vi "Two Parameter Marco Reparam.vi"() -> ()   [LabVIEW 2015]
uses:
  <vilib>/Platform/TimedLoop/XDataNode/timing_clust.ctl
  <vilib>/Platform/TimedLoop/XDataNode/nitl_modes.ctl
  <vilib>/Platform/TimedLoop/XDataNode/wakeup.ctl
  <vilib>/DAQmx/read.llb/DAQmx Read (Analog DBL 1Chan 1Samp).vi
  <vilib>/DAQmx/read.llb/DAQmx Read (Analog 1D DBL NChan 1Samp).vi
  <vilib>/DAQmx/create/channels.llb/DAQmx Create Channel (AI-Voltage-Basic).vi
  <vilib>/Enthought/Python Integration Toolkit/api/Unpack Double.vi
  <vilib>/DAQmx/miscellaneous.llb/DAQmx Fill In Error Info.vi
  <vilib>/Platform/TimedLoop/XDataNode/XDataNode.xnode
  Program Files/neMESYS_SDK/neMESYS LabVIEW Kit/neMESYS LabVIEW Integration Kit.lvlib
  <vilib>/Platform/TimedLoop/XDataNode/XDNodeRunTimeDep.lvlib
  Conor/Temp CN7500/Omega CN7500/Omega CN7500.lvlib
  <vilib>/Enthought/Python Integration Toolkit/Python Integration Toolkit.lvlib
panel:
  in  "LogFileName must end with .txt":string
  out "Param 1 8":dbl
  out "T value 1 8":dbl
  out "Param 2 8":dbl
  out "T value 2 8":dbl
  out "T Ref 8":dbl
  out "Correlation 8":dbl
  out "X2 8":dbl
  out "X2 ref 8":dbl
  out "Temp 9":dbl
  out "Flow 9":dbl
  out "Conc 9":dbl
  out "C BAcid 8":dbl
  out "C EB 8":dbl
  out "Exp 9":bool
  out "Param 1 7":dbl
  out "T value 1 7":dbl
  out "Param 2 7":dbl
  out "T value 2 7":dbl
  out "T Ref 7":dbl
  out "Correlation 7":dbl
  out "X2 7":dbl
  out "X2 ref 7":dbl
  out "Temp 8":dbl
  out "Flow 8":dbl
  out "Conc 8":dbl
  out "C BAcid 7":dbl
  out "C EB 7":dbl
  out "Exp 8":bool
  out "Param 1 6":dbl
  out "T value 1 6":dbl
  out "Param 2 6":dbl
  out "T value 2 6":dbl
  out "T Ref 6":dbl
  out "Correlation 6":dbl
  out "X2 6":dbl
  out "X2 ref 6":dbl
  out "Temp 7":dbl
  out "Flow 7":dbl
  out "Conc 7":dbl
  out "C BAcid 6":dbl
  out "C EB 6":dbl
  out "Exp 7":bool
  out "Param 1 5":dbl
  out "T value 1 5":dbl
  out "Param 2 5":dbl
  out "T value 2 5":dbl
  out "T Ref 5":dbl
  out "Correlation 5":dbl
  out "X2 5":dbl
  out "X2 ref 5":dbl
  out "Temp 6":dbl
  out "Flow 6":dbl
  out "Conc 6":dbl
  out "C BAcid 5":dbl
  out "C EB 5":dbl
  out "Exp 6":bool
  out "Param 1 4":dbl
  out "T value 1 4":dbl
  out "Param 2 4":dbl
  out "T value 2 4":dbl
  out "T Ref 4":dbl
  out "Correlation 4":dbl
  out "X2 4":dbl
  out "X2 ref 4":dbl
  out "Temp 5":dbl
  out "Flow 5":dbl
  out "Conc 5":dbl
  out "C BAcid 4":dbl
  out "C EB 4":dbl
  out "Exp 5":bool
  out "Param 1 3":dbl
  out "T value 1 3":dbl
  out "Param 2 3":dbl
  out "T value 2 3":dbl
  out "T Ref 3":dbl
  out "Correlation 3":dbl
  out "X2 3":dbl
  out "X2 ref 3":dbl
  out "Temp 4":dbl
  out "Flow 4":dbl
  out "Conc 4":dbl
  out "C BAcid 3":dbl
  out "C EB 3":dbl
  out "Exp 4":bool
  out "Conc 3":dbl
  out "Flow 3":dbl
  out "Temp 3":dbl
  in  "Design Criteria A or D or E or SV":string
  in  "Reparameterise? ON or OFF":string
  out "Exp 2":bool
  out "C EB 1":dbl
  out "C BAcid 1":dbl
  out "X2 ref 2":dbl
  out "X2 2":dbl
  out "Exp 2":bool
  out "Liquid Inlet Pressure (bar g)":dbl
  in  "Liquid P sensor Terminal Configuration":i32(ring)=-1 items=["default"=-1, "RSE"=10083, "NRSE"=10078, "Differential"=10106, "Pseudodifferential"=12529]
  in  "Liquid P sensor Physical Channel":tag="Dev1/ai0"
  in  "Temp 2":dbl
  in  "Conc 2":dbl
  in  "Flow 2":dbl
  out "Correlation 2":dbl
  out "T Ref 2":dbl
  out "Exp 3":bool
  out "Exp 1":bool
  out "Exp 0":bool
  out "Conc 1":dbl
  out "Flow 1":dbl
  out "Temp 1":dbl
  out "Conc 2":dbl
  out "Flow 2":dbl
  out "Temp 2":dbl
  out "Param 1 2":dbl
  out "T value 1 2":dbl
  out "Param 2 2":dbl
  out "T value 2 2":dbl
  out "C BAcid 2":dbl
  out "C EB 2":dbl
  in  "Result file name must end with .xlsx":string
  in  "HPLC file Name, dont need extension":string
  out "Desired Conc Not Possible":bool
  in  "Safety or Emergency Syringe Control":bool
  out "Feed Concentration (M)":dbl
  out "Total Flowrate (uL/min)":dbl
  out "Gas Back Pressure (barg)":dbl
  in  "Shut down in empty?\nLeft off, right on":bool
  in  "Clear":bool
  out "Safety Shut Down Pressure (barg)":dbl
  out "Calculated Pressure":dbl[](graph)
  out "Safety Shut Down Temp":dbl
  out "Actual Temp (oC)":dbl
  out "Temperature":dynamicdata(graph)
  out "Temp Set Point (oC)":dbl
  in  "Temp 1":dbl
  in  "Temp 0":dbl
  in  "Update Temperature Set Point":bool
  in  "Automated Experiments or Direct Control":bool
  in  "Set Point (oC)":dbl
  out "loop ind":dbl
  in  "Stop everything":bool
  in  "Skip Exp":bool
  in  "Minutes between Exp":dbl min=0.0 step=0.05
  in  "Refill 4":bool
  in  "Refill 3":bool
  in  "Refill 2":bool
  in  "Refill 1":bool
  in  "Empty 4":bool
  in  "Empty 3":bool
  in  "Empty 2":bool
  in  "Empty 1":bool
  in  "Calibrate 4":bool
  in  "Calibrate 3":bool
  in  "Calibrate 2":bool
  in  "Calibrate 1":bool
  in  "Stop Dose 4":bool
  in  "Stop Dose 3":bool
  in  "Stop Dose 2":bool
  in  "Stop Dose 1":bool
  in  "Flow 1":dbl
  in  "Conc 1":dbl
  in  "Flow 0":dbl
  in  "Conc 0":dbl
  in  "Generate Flow":bool
  in  "Set Flowrate 1":dbl
  in  "Set Flowrate 2":dbl
  in  "Set Flowrate 3":dbl
  in  "Set Flowrate 4":dbl
  in  "High Conc":dbl min=0.0 max=2.0
  in  "Low Conc":dbl min=0.0 max=2.0
  out "Volumetric Fraction Acid":dbl min=0.0 max=1.0
  out "Syringe Level 4":dbl(slide) scale=0.0..5500.0
  out "Syringe Level 3":dbl(slide) scale=0.0..5500.0
  out "Syringe Level 2":dbl(slide) scale=0.0..5500.0
  out "Syringe Level 1":dbl(slide) scale=0.0..5500.0
  out "Flowrate 4 Ethanol":dbl
  out "Flowrate 3 Acid":dbl
  out "Flowrate 2 High":dbl
  out "Flowrate 1 Low":dbl
  # "Pre Planned Experiments"
  # "Conducted Experiments Set Points"
  # "Safety (start and end)"
  # "Current Conditions"
  # "(uL/min)"
  # "Coerced to nearest possible"
  # "Experimental Info"
  # "Acid must be between 0 and 1, normally 0.1 for 10%"
  # "Direct Control"
  # "Unit of Gas Flow NmL/min"
  # "I swapped syringe 1 and 2, so now 2 is high and 1 is low"
  # "Emergency Syringe Control Below"
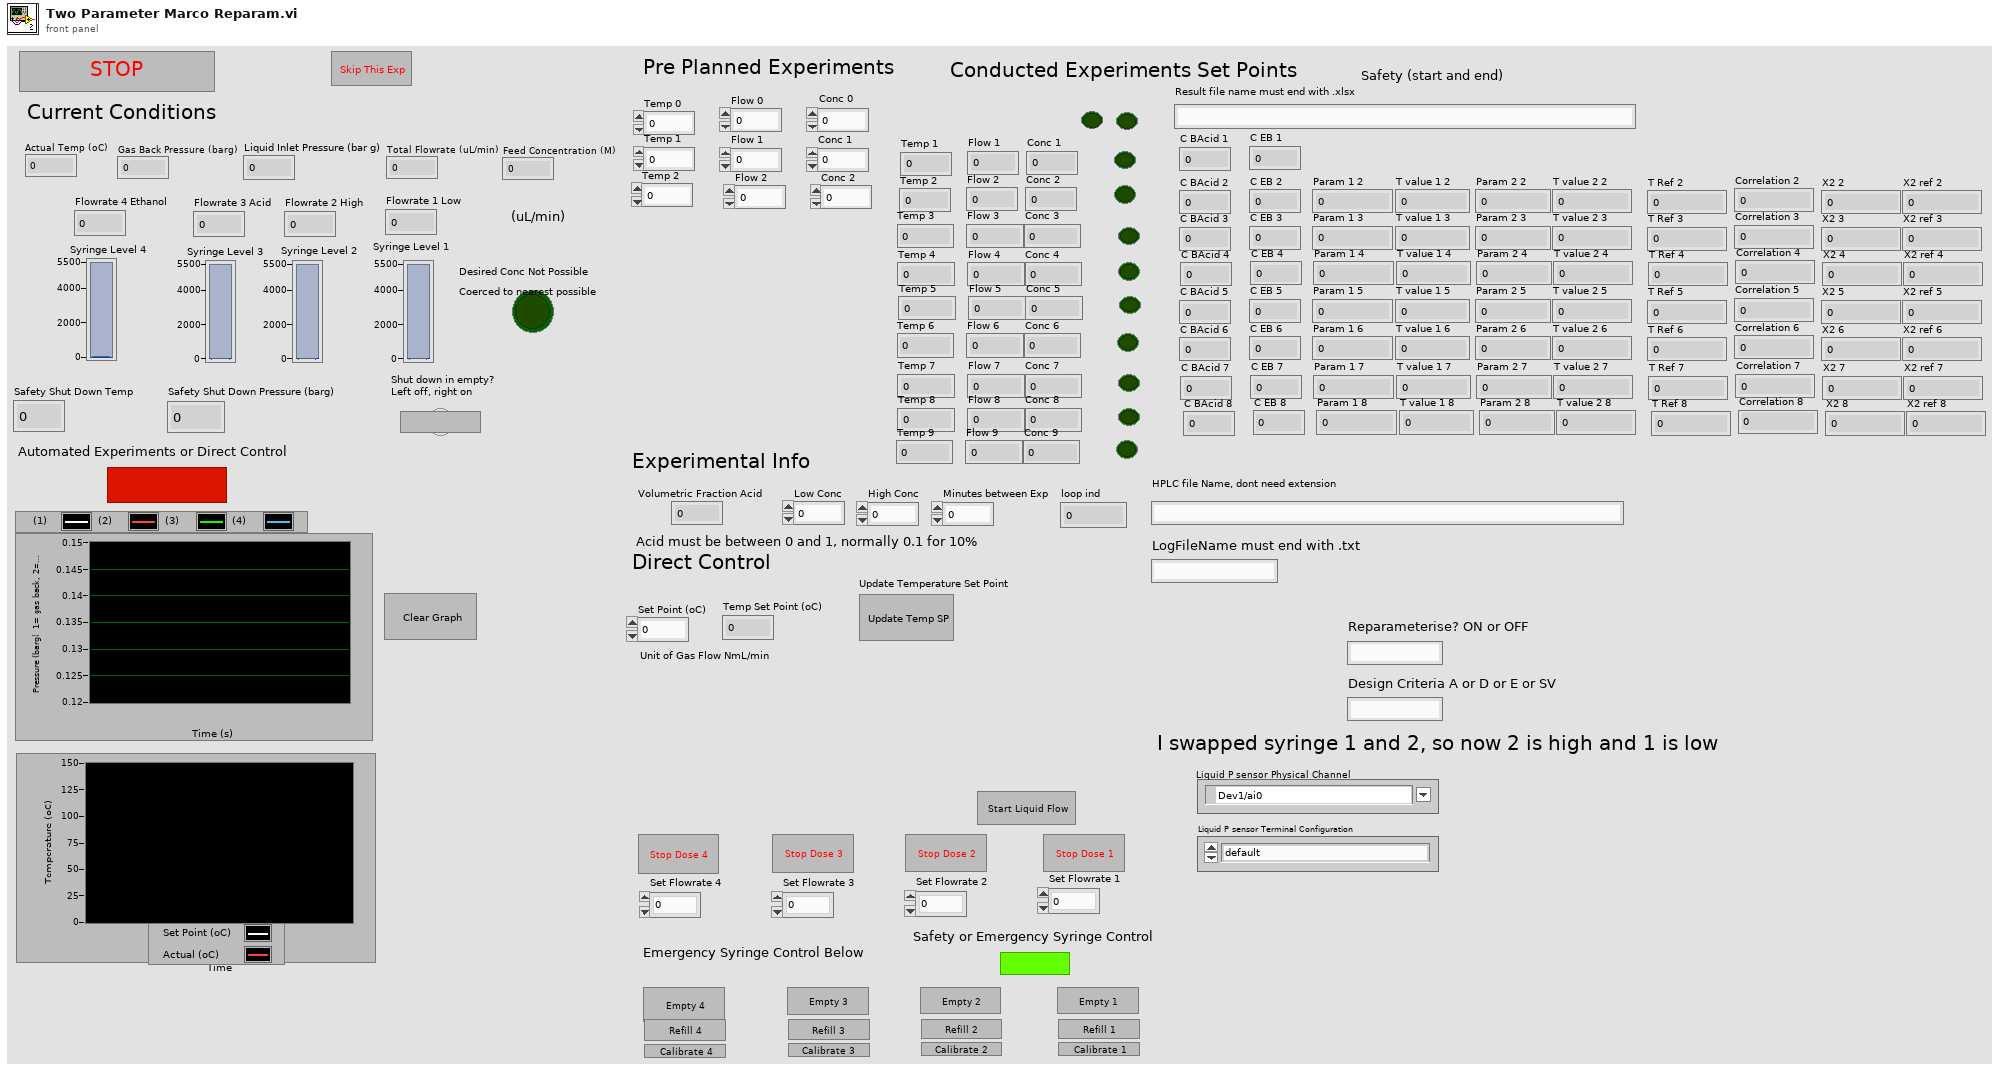
[diagram p1: front panel]
types:
  T1 = typedef "XDNodeRunTimeDep.lvlib/timing_clust.ctl" = cluster{"Expected End [f-1]":u64, "Actual End [f-1]":u64, "Finished Late? [f-1]":bool, "Expected End [i-1]":u64, "Actual End [i-1]":u64, "Finished Late? [i-1]":bool, "Expected Start [i]":u64, "Actual Start [i]":u64, "Expected Start [f]":u64, "Actual Start [f]":u64, "Source Name":string, "Structure Name":string, "Period":i64, "Deadline":i64, "Offset":i64, "Start":i64, "Priority":i32, "Timeout":i32, "Mode":T2, "Wakeup Reason":T3, "Error":errorcluster, "Source Type":string, "Secondary Source Type":string, "Global End Time":u64, "Global Start Time":u64, "Frame Duration":u64, "Iteration Duration":u64, "Assigned CPU":i32, "I/O Scan Engine Mode":u32}
  T2 = typedef "XDNodeRunTimeDep.lvlib/nitl_modes.ctl" = enum32{"No Change", "Process missed periods, maintain original phase", "Discard missed periods, maintain original phase", "Process missed periods, ignore original phase", "Discard missed periods, ignore original phase"}
  T3 = typedef "XDNodeRunTimeDep.lvlib/wakeup.ctl" = enum32{"Normal", "Aborted", "Asynchronous wakeup", "Timing source error", "Timed loop error", "Timeout"}
  T4 = typedef "Python Integration Toolkit.lvlib/Session ID.ctl" = u64
  T5 = typedef "Python Integration Toolkit.lvlib/Python Objects.ctl" = variant
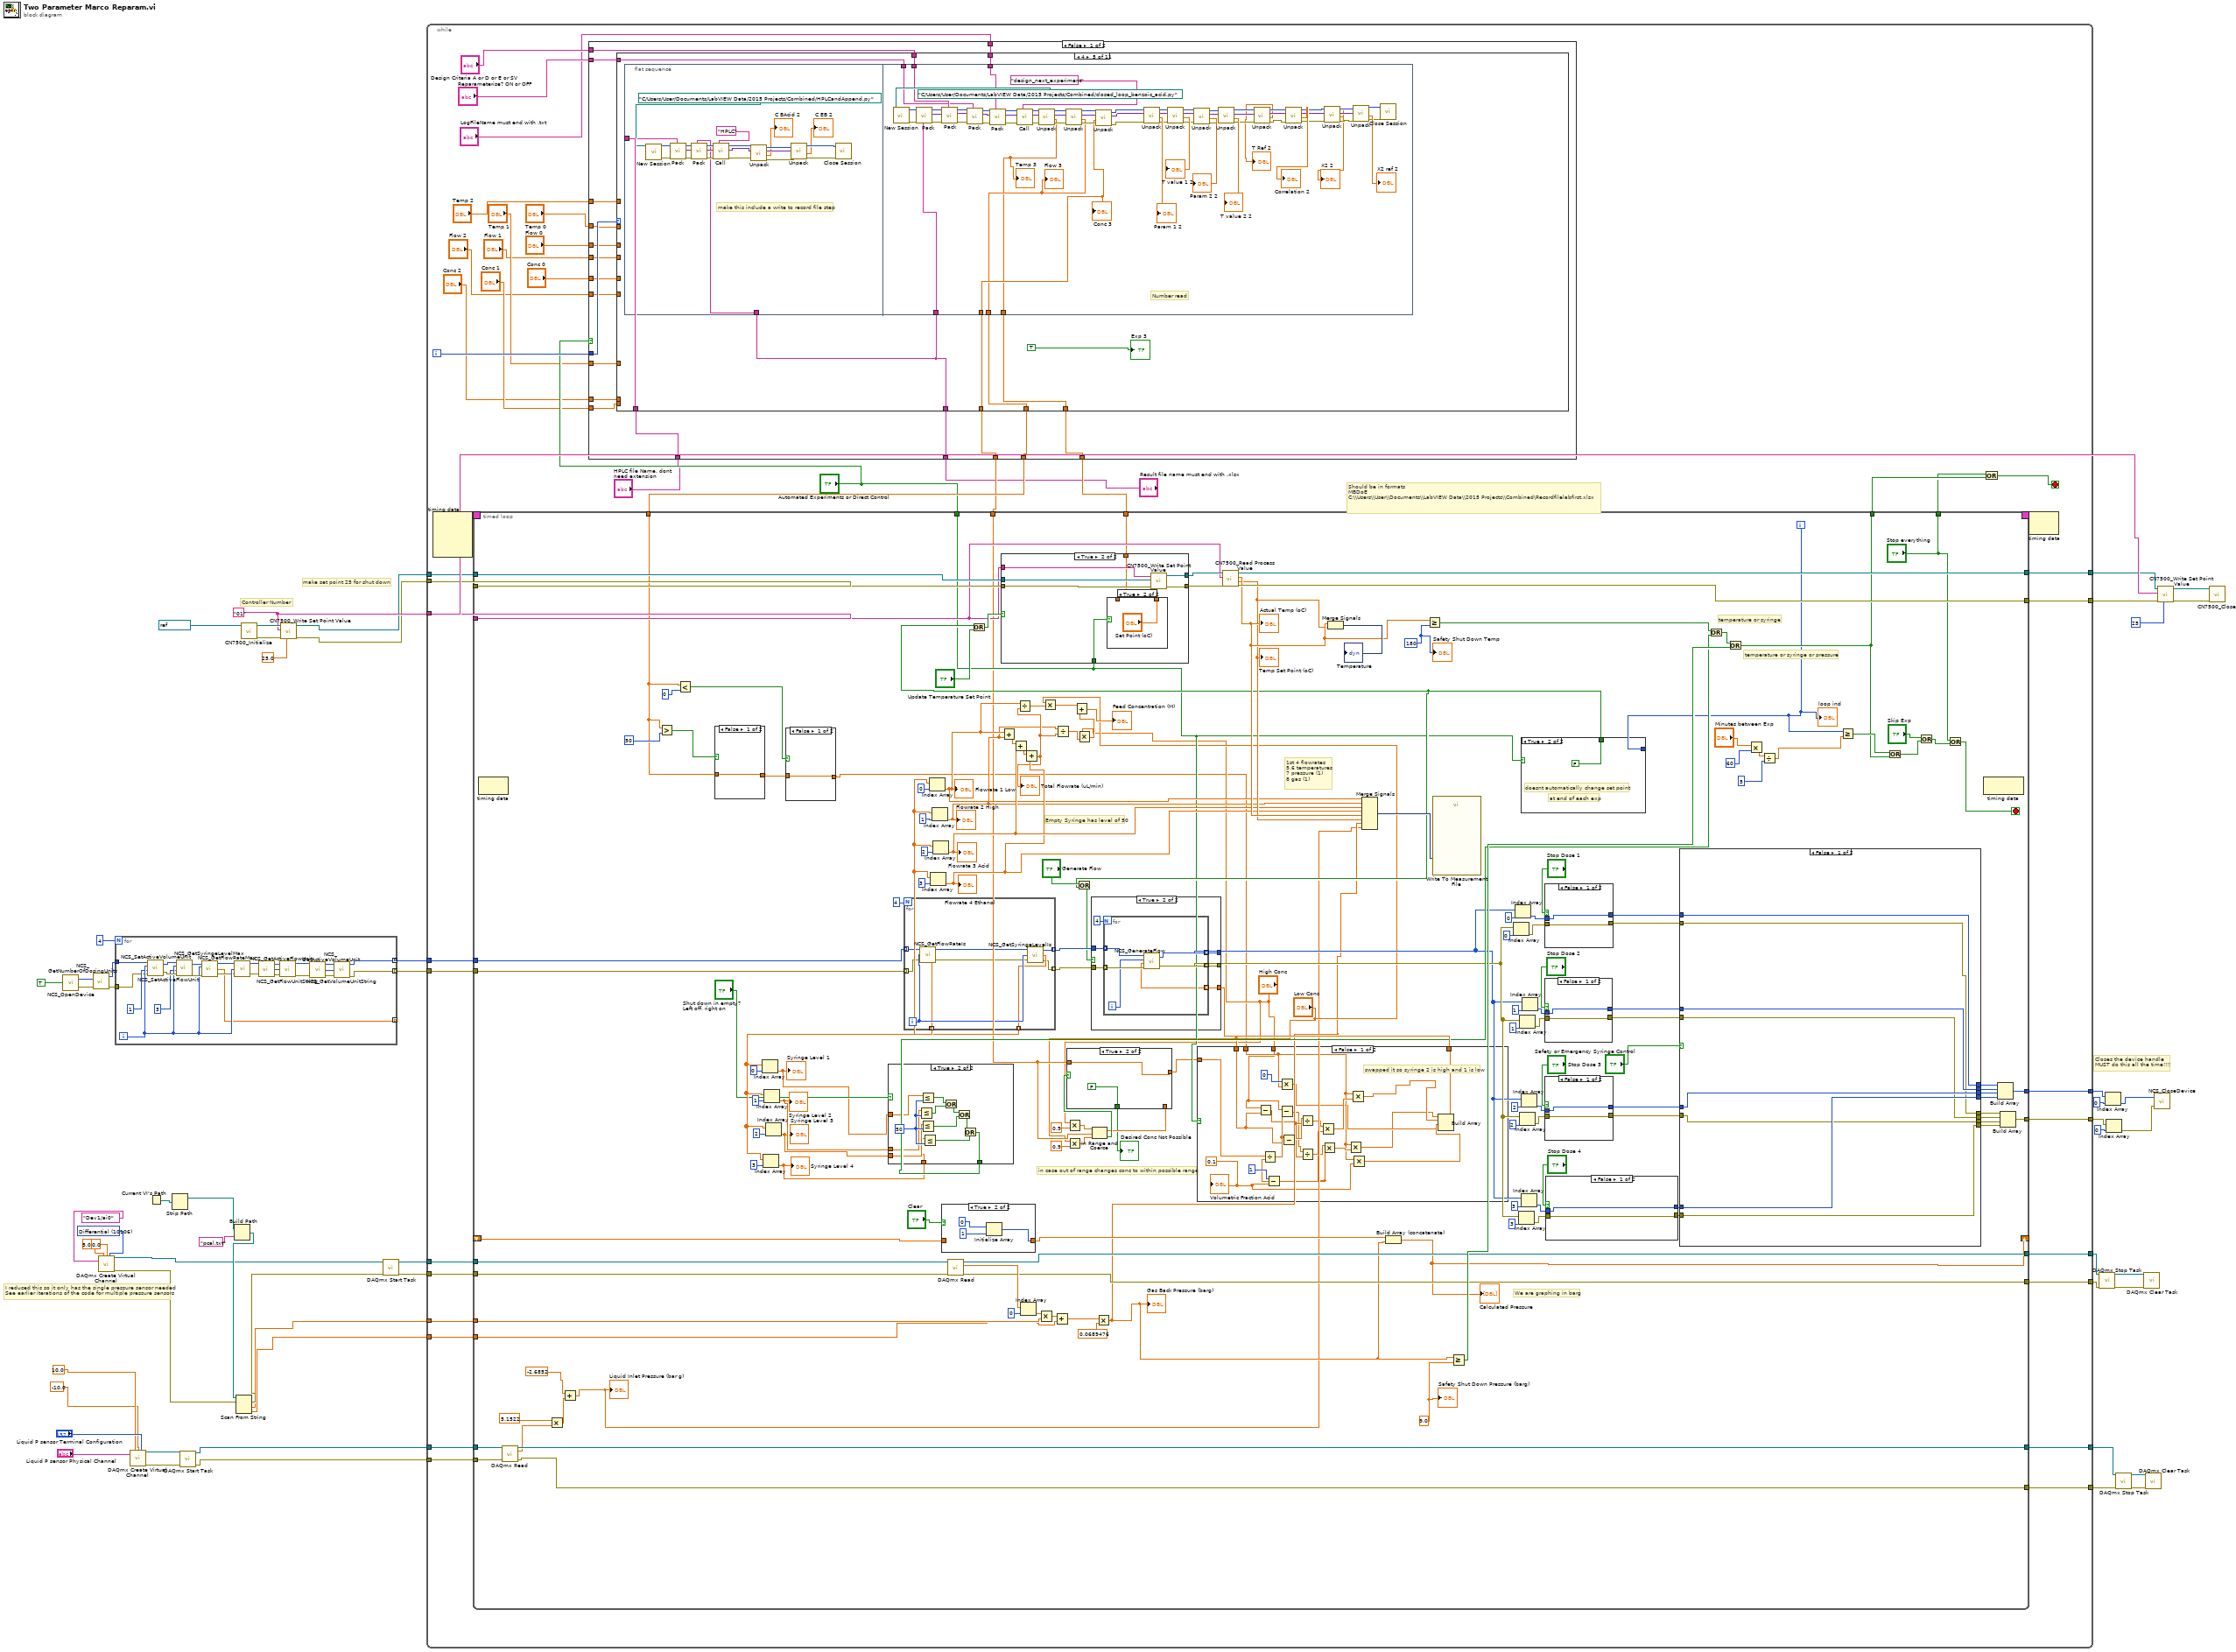
[diagram p0: block diagram]
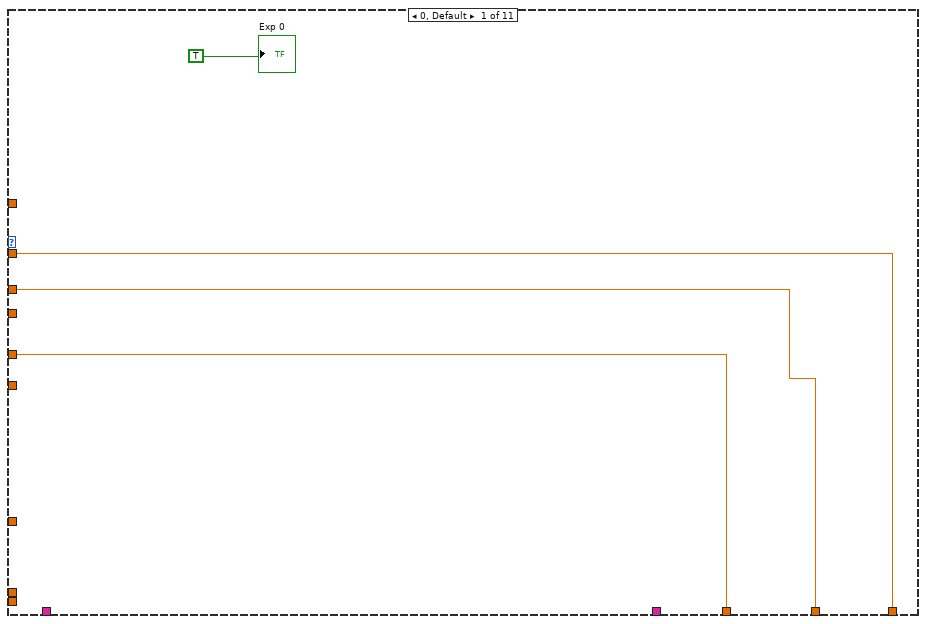
[diagram p2: hidden frame]
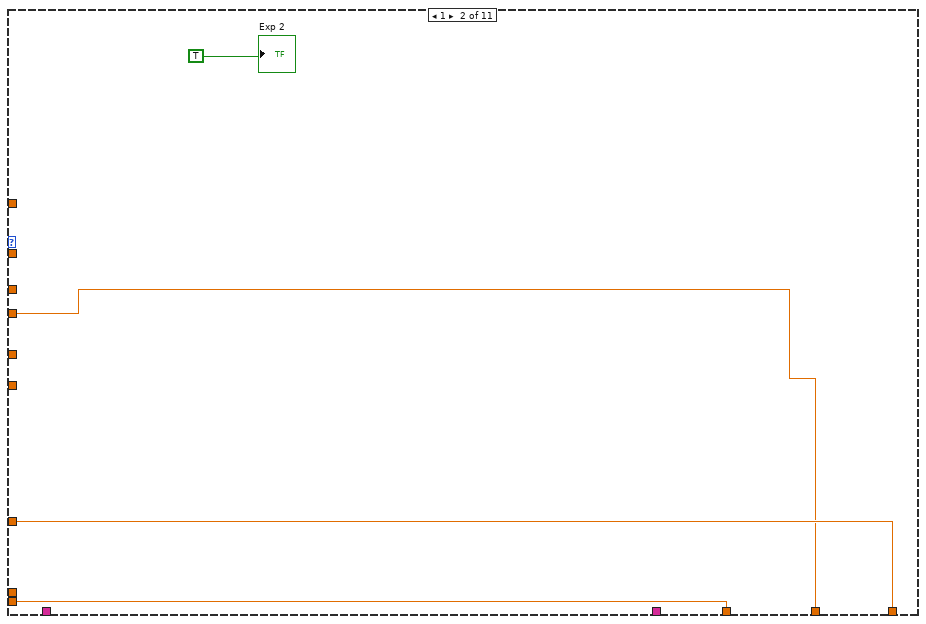
[diagram p3: hidden frame]
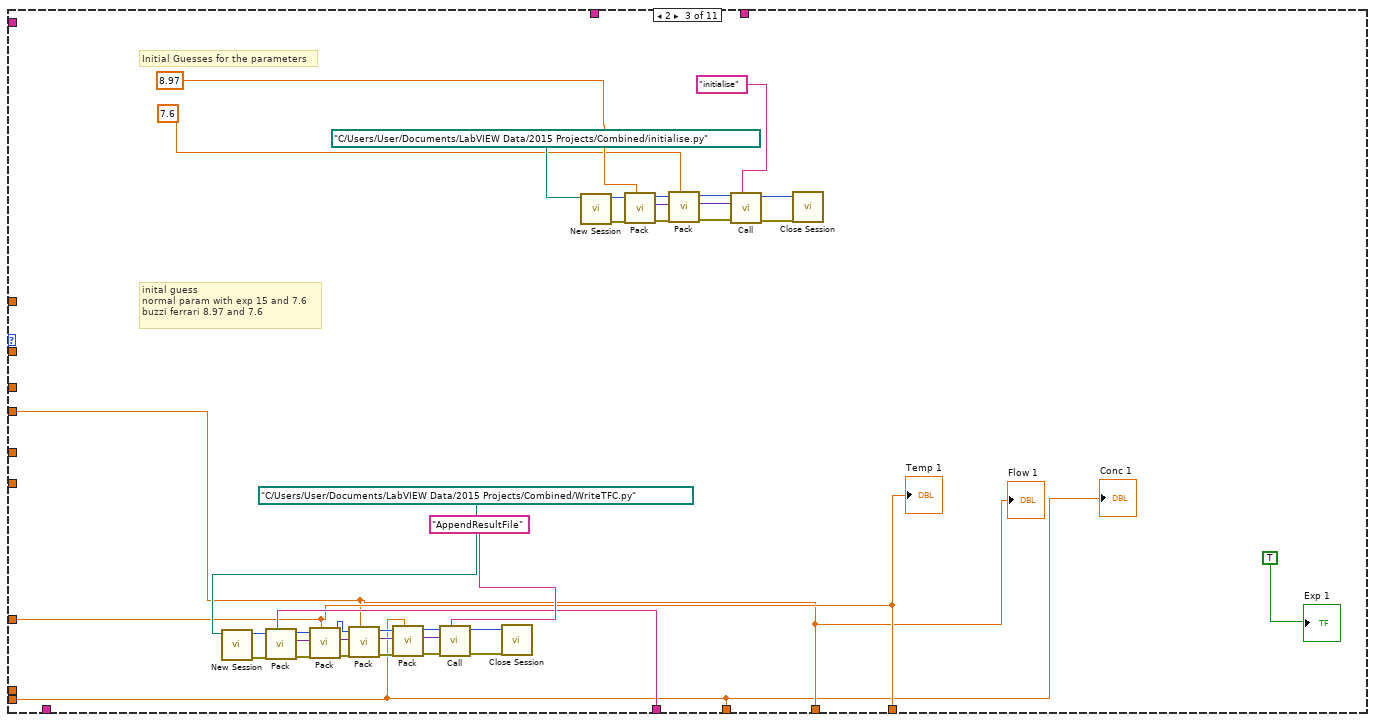
[diagram p4: hidden frame]
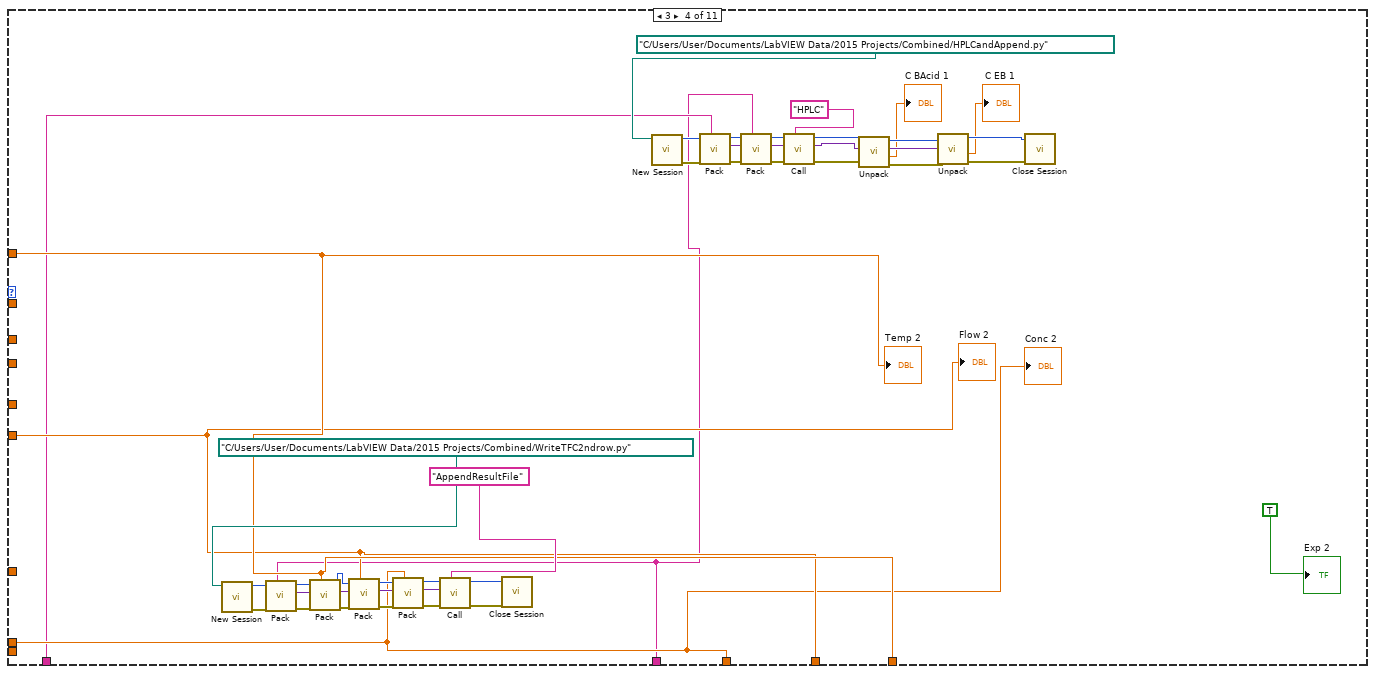
[diagram p5: hidden frame]
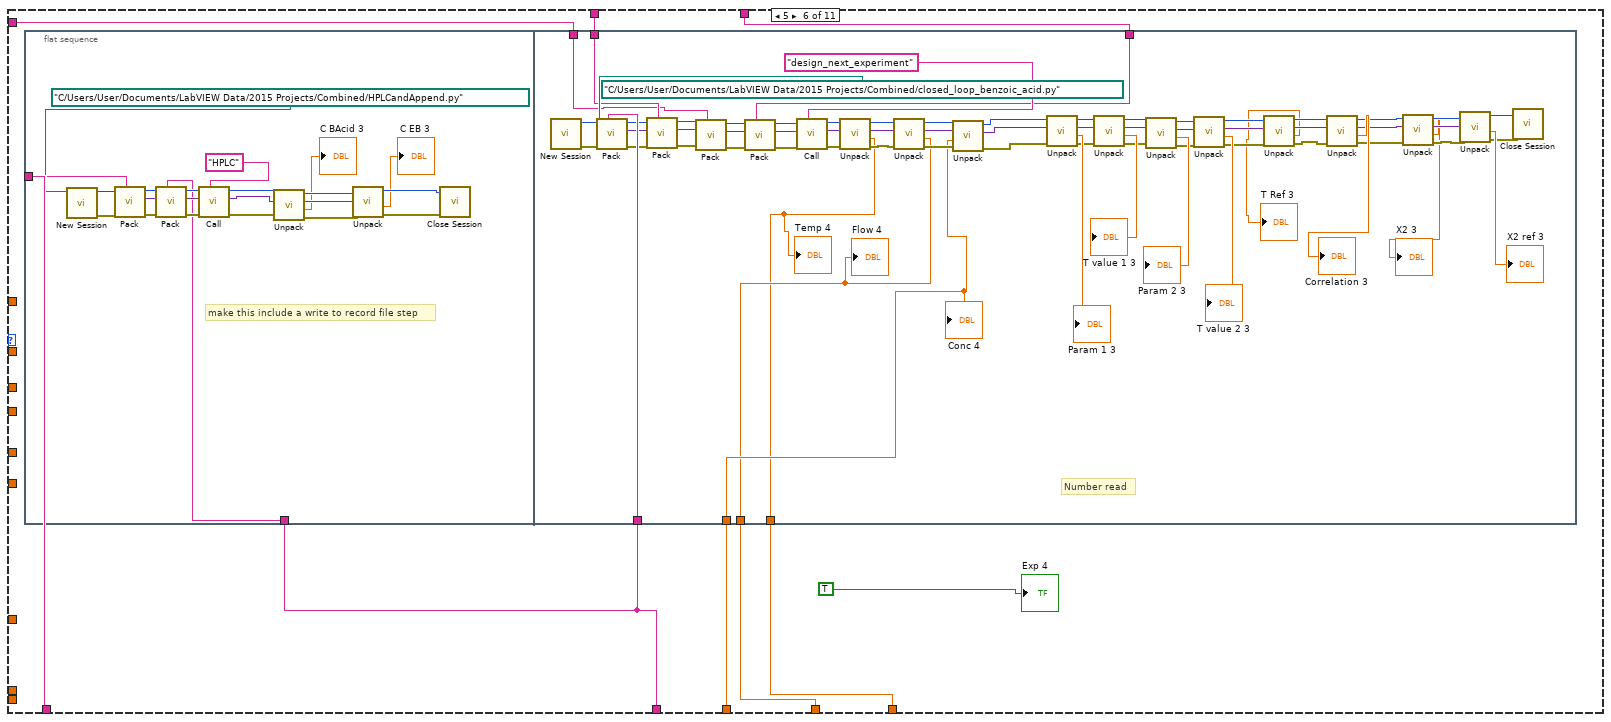
[diagram p6: hidden frame]
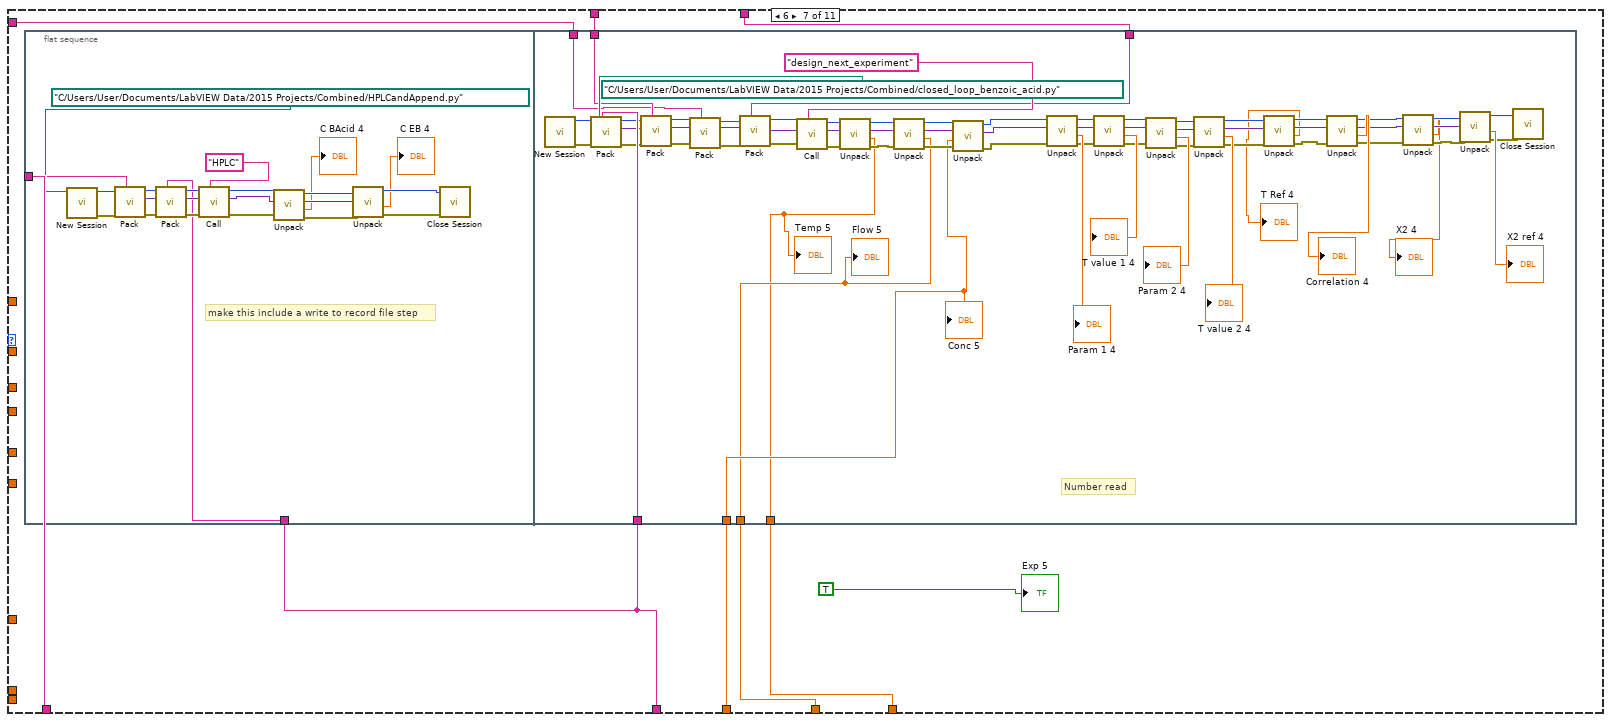
[diagram p7: hidden frame]
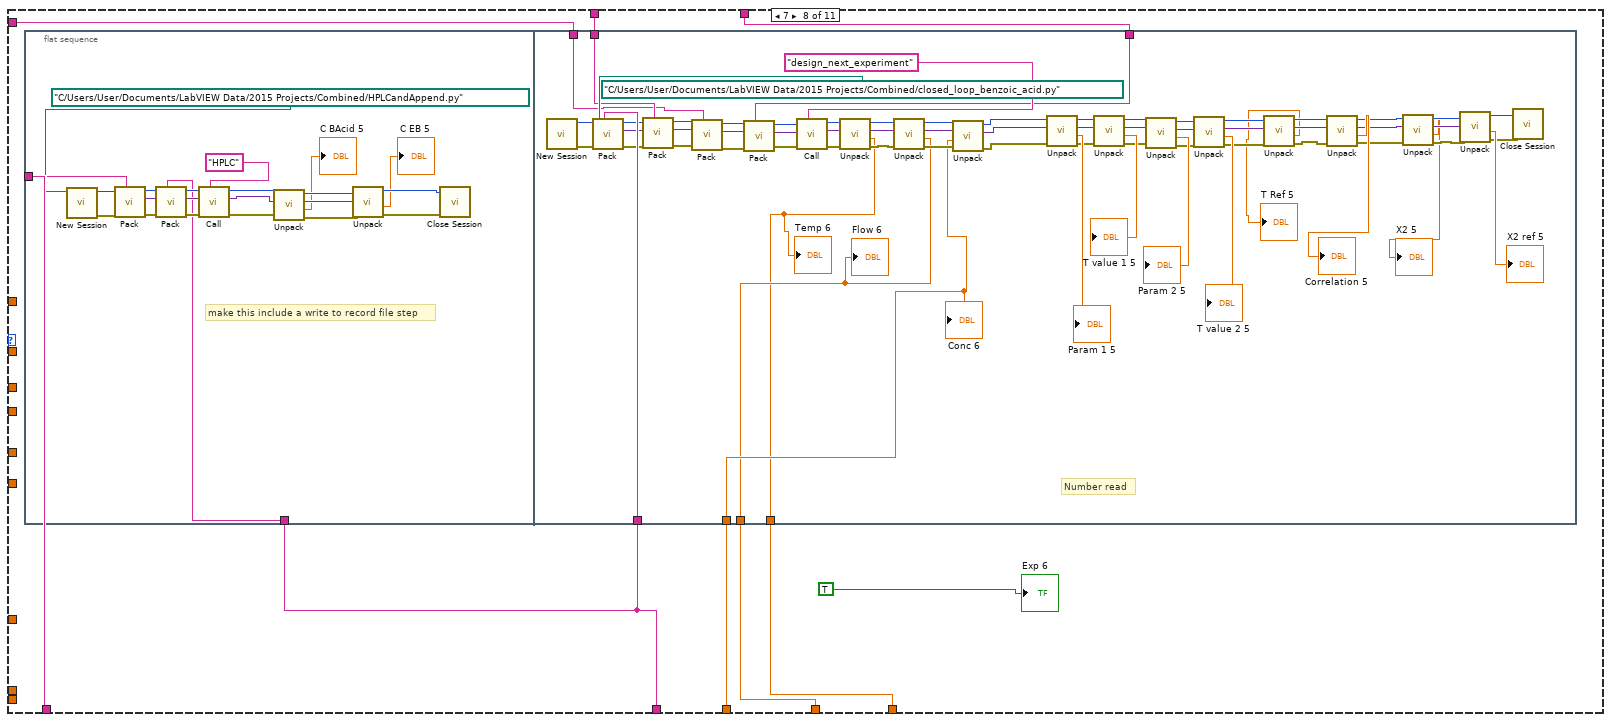
[diagram p8: hidden frame]
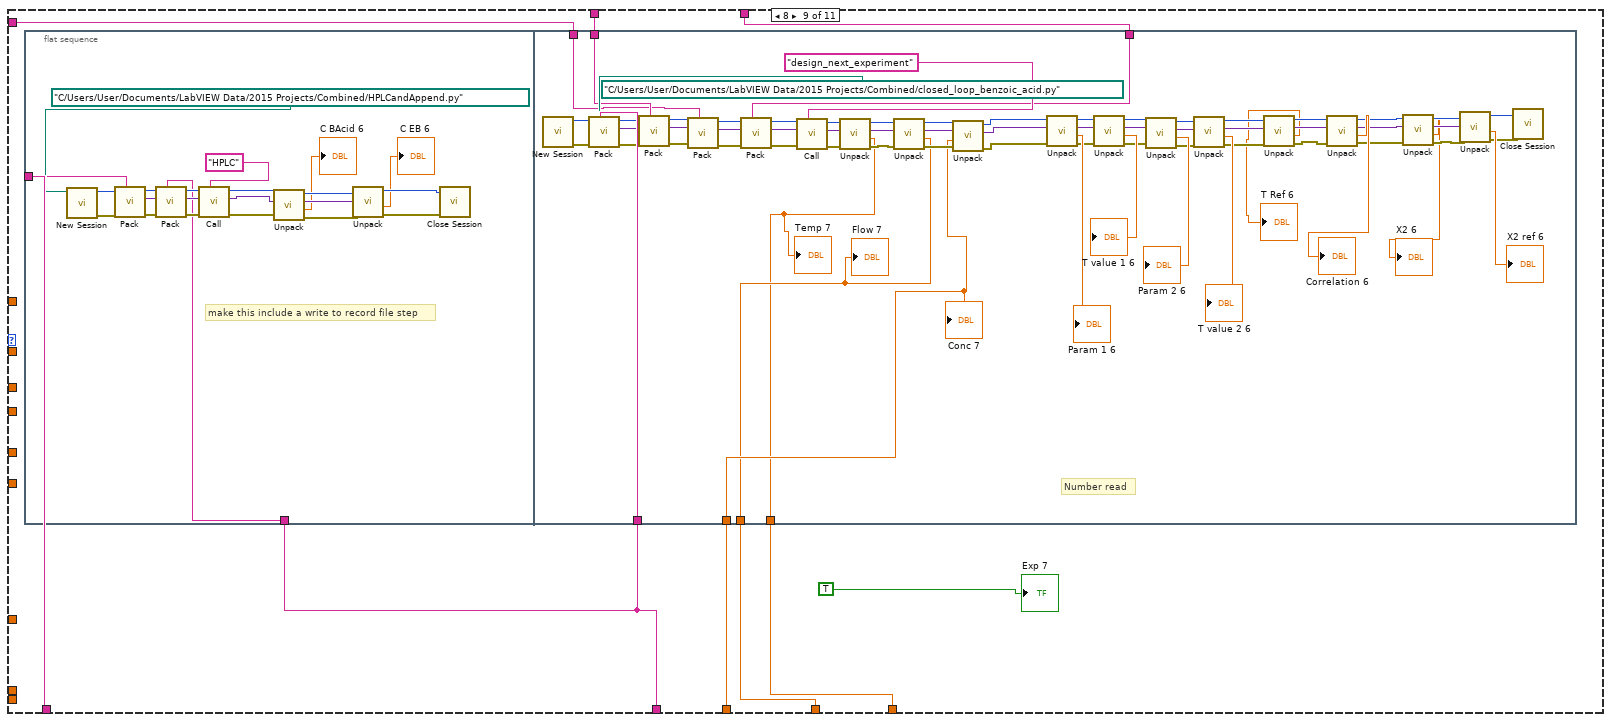
[diagram p9: hidden frame]
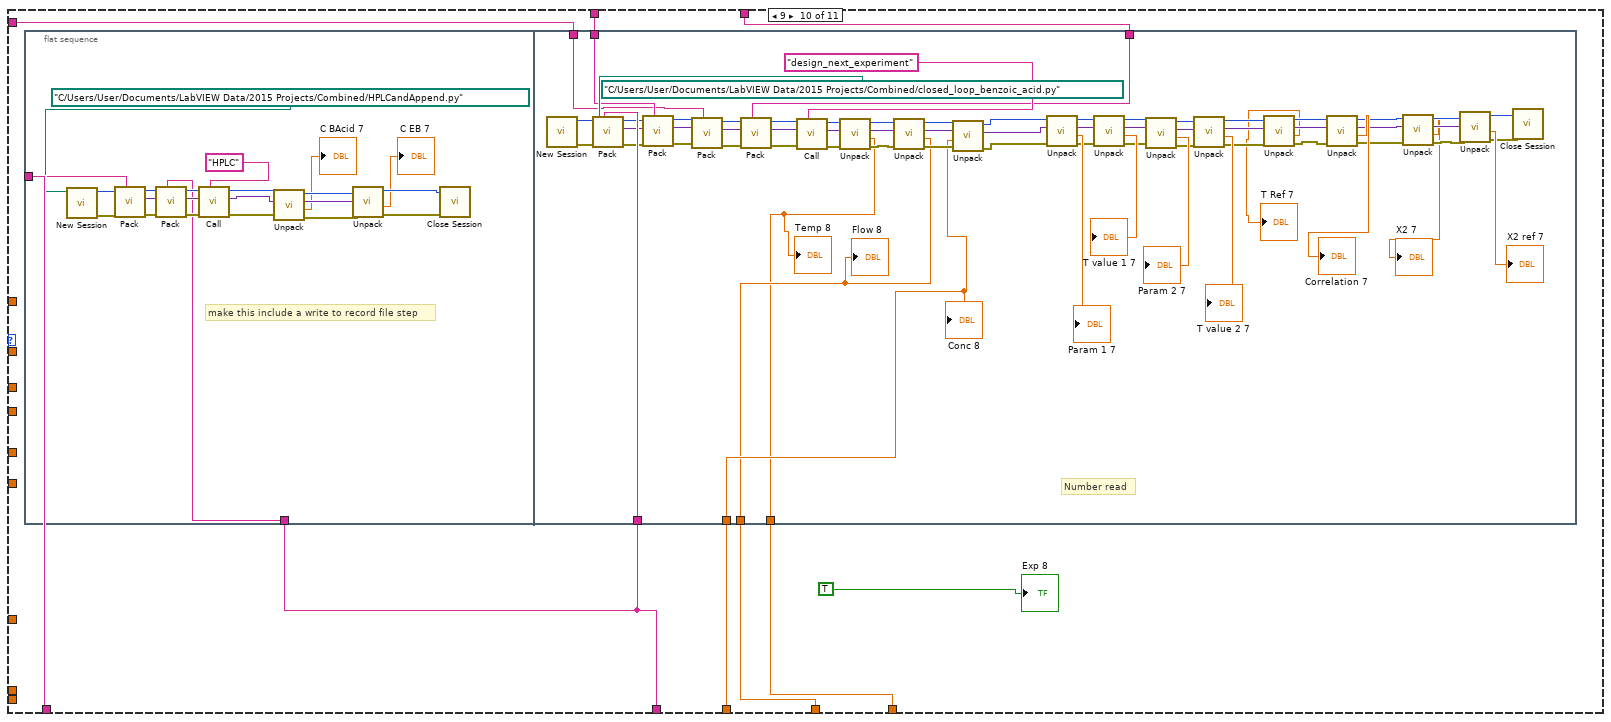
[diagram p10: hidden frame]
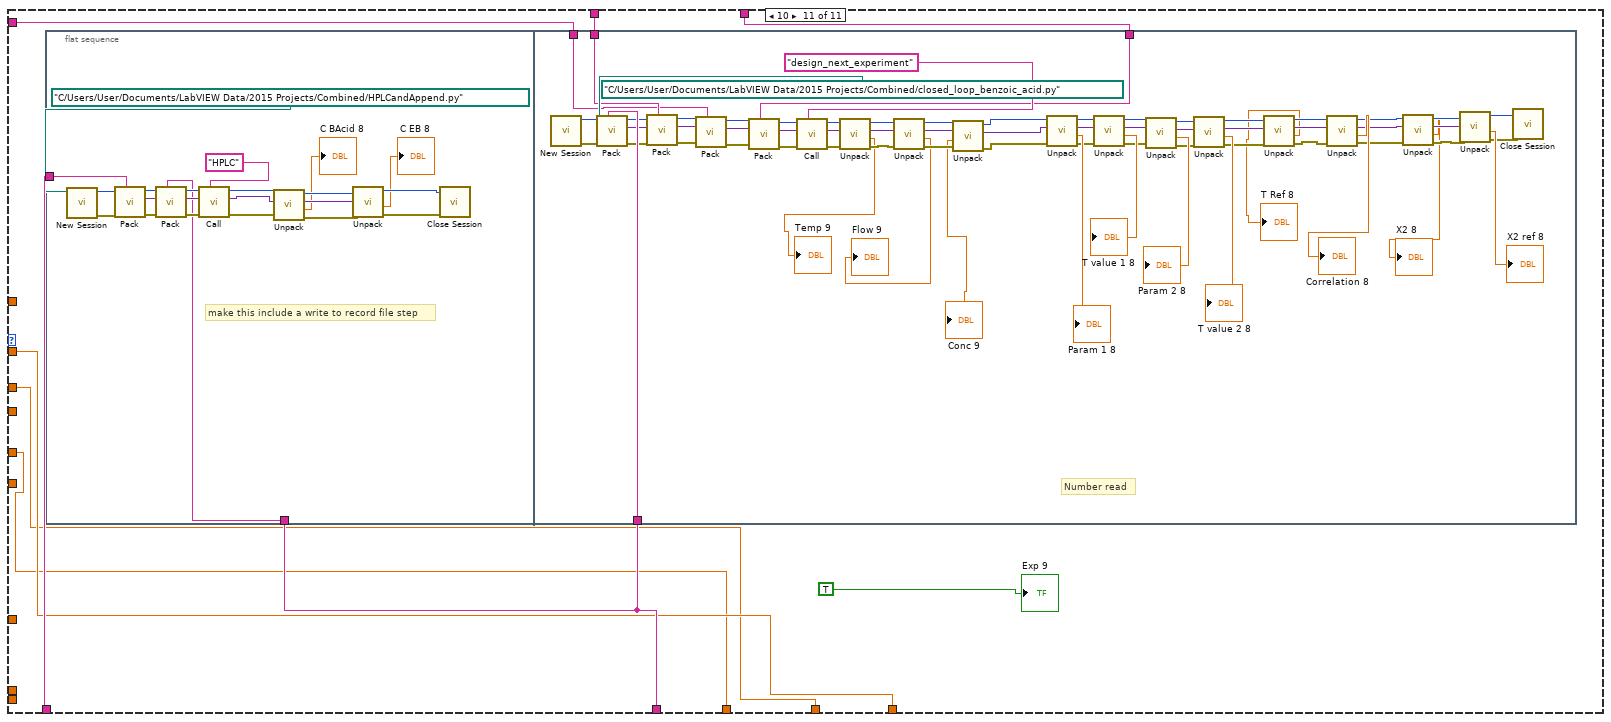
[diagram p11: hidden frame]
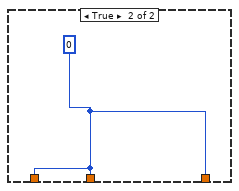
[diagram p12: hidden frame]
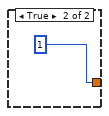
[diagram p13: hidden frame]
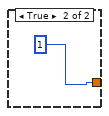
[diagram p14: hidden frame]
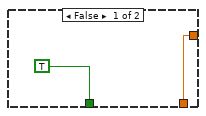
[diagram p15: hidden frame]
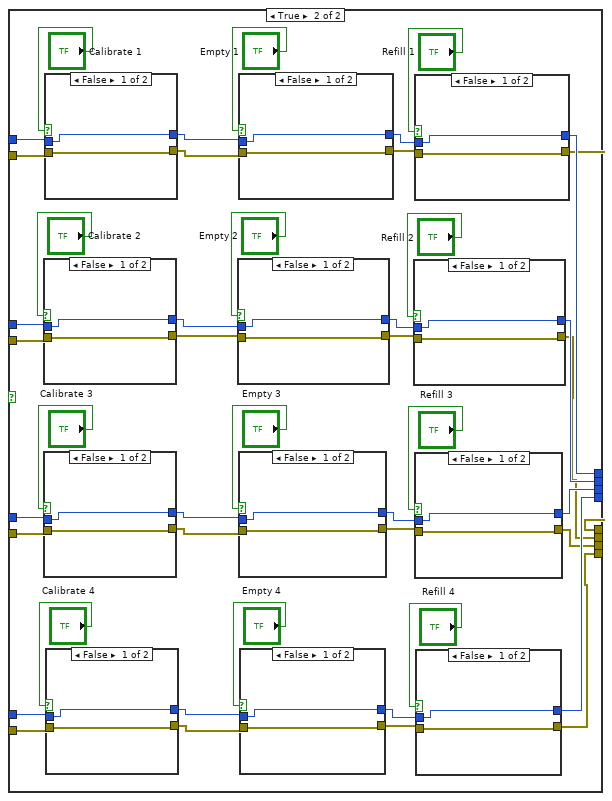
[diagram p16: hidden frame]
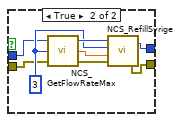
[diagram p17: hidden frame]
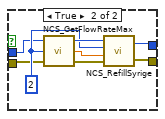
[diagram p18: hidden frame]
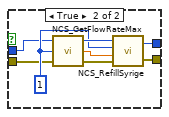
[diagram p19: hidden frame]
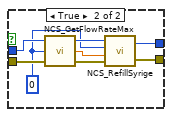
[diagram p20: hidden frame]
diagram:
  w29 = 10106 items=["default"=-1, "RSE"=10083, "NRSE"=10078, "Differential"=10106, "Pseudodifferential"=12529] ("input terminal configuration")
  w36 = "01" ("Controller Number")
  # "I reduced this so it only has the single pressure sensor needed\nSee earlier iterations of the code for multiple pressure sensors"
  # "make set point 25 for shut down"
  # "Controller Number"
  # "Closes the device handle \nMUST do this all the time!!!!"
  n1 = call "NCS_OpenDevice.vi"("show status window"=TRUE) -> ("device handle"=w55:u32, "error out"=w54:errorcluster)
  n2 = call "NCS_GetNumberOfDosingUnits.vi"("device handle in"=w55, "error in (no error)"=w54) -> ("device handle out"=w52:u32, "error out"=w53:errorcluster)  [unwired: 1 out]
  n3 = call-poly <vilib>:"DAQmx Create Virtual Channel.vi"("maximum value"=5.0, "minimum value"=0.0, "input terminal configuration"=w29, "physical channels"=tag "Dev1/ai0") -> ("task out"=w13:refnum<k21>, "error out"=w14:errorcluster)  [unwired: 10 in]
  n4 = for {
    N: 4 -> [_]
    tunnel: [w61] -> w51 mode=indexing
    tunnel: [w60] -> w50 mode=indexing
    tunnel: [w74] -> _ mode=indexing
    tunnel: w53 -> [w59]
    tunnel: w52 -> [w58]
    i -> [w77]
    n5 = call "NCS_SetActiveVolumeUnit.vi"("error in (no error)"=w59, "active volume unit"=1, "dosingunit"=w77, "device handle in"=w58) -> ("error out"=w80:errorcluster, "device handle out"=w81:u32)
    n6 = call "NCS_SetActiveFlowUnit.vi"("error in (no error)"=w80, "active flow unit"=3, "dosingunit"=w77, "device handle in"=w81) -> ("error out"=w78:errorcluster, "device handle out"=w79:u32)
    n7 = call "NCS_GetSyringeLevelMax.vi"("error in (no error)"=w78, "dosingunit"=w77, "device handle in"=w79) -> ("error out"=w75:errorcluster, "syringe level max"=w74:dbl, "device handle out"=w76:u32)  [unwired: 1 out]
    n8 = call "NCS_GetFlowRateMax.vi"("error in (no error)"=w75, "dosingunit"=w77, "device handle in"=w76) -> ("error out"=w62:errorcluster, "device handle out"=w63:u32)  [unwired: 1 out]
    n9 = call "NCS_GetActiveFlowUnit.vi"("error in (no error)"=w62, "device handle in"=w63) -> ("error out"=w70:errorcluster, "active flow unit"=w69:u8, "device handle out"=w71:u32)  [unwired: 1 in]
    n10 = call "NCS_GetFlowUnitString.vi"("device handle in"=w71, "flow unit id"=w69, "error in (no error)"=w70) -> ("device handle out"=w66:u32, "error out"=w65:errorcluster)  [unwired: 2 out]
    n11 = call "NCS_GetActiveVolumeUnit.vi"("error in (no error)"=w65, "device handle in"=w66) -> ("error out"=w67:errorcluster, "active volume unit"=w68:u8, "device handle out"=w64:u32)  [unwired: 1 in]
    n12 = call "NCS_GetVolumeUnitString.vi"("device handle in"=w64, "volume unit id"=w68, "error in (no error)"=w67) -> ("device handle out"=w61:u32, "error out"=w60:errorcluster)  [unwired: 2 out]
  }
  n13 = call-poly <vilib>:"DAQmx Create Virtual Channel.vi"("maximum value"=10.0, "minimum value"=-10.0 ("maximum value"), "input terminal configuration"="Liquid P sensor Terminal Configuration", "physical channels"="Liquid P sensor Physical Channel") -> ("task out"=w9:refnum<k21>, "error out"=w10:errorcluster)  [unwired: 10 in]
  n14 = Current VI's Path() -> (path=w27:path)
  n15 = Strip Path(path=w27) -> (stripped path=w25:path)  [unwired: 1 out]
  n16 = call <vilib>:"DAQmx Start Task.vi"("task/channels in"=w9, "error in"=w10) -> ("task out"=w8:refnum<k21>, "error out"=w7:errorcluster)  [unwired: 12 in]
  n17 = Build Path(base path=w25, name or relative path="pcal.txt") -> (appended path=w26:path)
  n18 = Scan From String(w26, w14) -> (w23:errorcluster, output 1=w20:dbl, output 2=w19:dbl)  [unwired: 3 in, 1 out]
  n19 = call "CN7500_Initialize.vi"("VISA resource name"=refnum<visa-resource-name> "COM8") -> ("error out"=w42:errorcluster, "VISA resource name out"=w43:refnum<visa-resource-name>)  [unwired: 9 in]
  n20 = call "CN7500_Write Set Point Value.vi"("Target Set Point Value"=25.0, "error in (no error)"=w42, "Controller Number"=w36, "VISA In"=w43) -> ("error out"=w34:errorcluster, "VISA Out"=w35:refnum<visa-resource-name>)  [unwired: 6 in]
  n21 = call <vilib>:"DAQmx Start Task.vi"("task/channels in"=w13, "error in"=w23) -> ("task out"=w22:refnum<k21>, "error out"=w21:errorcluster)  [unwired: 12 in]
  n22 = while {
    tunnel: w51 -> [w124]
    tunnel: w50 -> [w123]
    tunnel: [w122] -> w45
    tunnel: [w121] -> w44
    tunnel: w36 -> [w118]
    tunnel: w35 -> [w117]
    tunnel: w34 -> [w116]
    tunnel: [w115] -> w33
    tunnel: [w114] -> w32
    tunnel: w22 -> [w112]
    tunnel: w21 -> [w111]
    tunnel: w20 -> [w110]
    tunnel: w19 -> [w109]
    tunnel: [w108] -> w16
    tunnel: [w107] -> w15
    tunnel: w8 -> [w91]
    tunnel: w7 -> [w90]
    tunnel: [w89] -> w5
    tunnel: [w88] -> w3
    i -> [w101]
    stop <- w106 stop-if-true
    # "Should be in formats \nMBDoE\nC:\\\\Users\\\\User\\\\Documents\\\\LabVIEW Data\\\\2015 Projects\\\\Combined\\Recordfilelabfirst.xlsx"
    n23 = node-c288() -> (w120:T1)  [unwired: 4 in]
    n24 = case shown="False" "Automated Experiments or Direct Control" {
      tunnel: [w139 w911] -> w104
      tunnel: [w137 w911] -> w103
      tunnel: [w141 w911] -> w102
      tunnel: w101 -> [w142 _]
      tunnel: "Conc 0" -> [w140 _]
      tunnel: "Flow 0" -> [w136 _]
      tunnel: "Temp 0" -> [w138 _]
      tunnel: "Temp 1" -> [w134 _]
      tunnel: "Flow 1" -> [w133 _]
      tunnel: "Conc 1" -> [w132 _]
      tunnel: "HPLC file Name, dont need extension" -> [w131 _]
      tunnel: "Result file name must end with .xlsx" -> [w135 _]
      tunnel: "Temp 2" -> [w130 _]
      tunnel: "Flow 2" -> [w129 _]
      tunnel: "Conc 2" -> [w128 _]
      tunnel: "Design Criteria A or D or E or SV" -> [w127 _]
      tunnel: "Reparameterise? ON or OFF" -> [w126 _]
      tunnel: "LogFileName must end with .txt" -> [w125 _]
      frame False {
        n25 = case shown="4" w142 {
          tunnel: [w144 w147 w166 w210 w235 w332 w429 w526 w623 w720 w815] -> w141
          tunnel: w140 -> [w144 _ _ _ _ _ _ _ _ _ w815]
          tunnel: [w146 w149 w168 w212 w233 w330 w427 w524 w621 w718 w817] -> w139
          tunnel: w138 -> [w146 _ _ _ _ _ _ _ _ _ w817]
          tunnel: [w145 w148 w167 w211 w234 w331 w428 w525 w622 w719 w816] -> w137
          tunnel: w136 -> [w145 _ _ _ _ _ _ _ _ _ w816]
          tunnel: w135 -> [_ _ w169 w188 w239 w336 w433 w530 w627 w724 w821]
          tunnel: w134 -> [_ w149 w168 _ _ _ _ _ _ _ _]
          tunnel: w133 -> [_ w148 w167 _ _ _ _ _ _ _ _]
          tunnel: w132 -> [_ w147 w166 _ _ _ _ _ _ _ _]
          tunnel: w131 -> [_ _ _ w189 w240 w337 w434 w531 w628 w725 w822]
          tunnel: w130 -> [_ _ _ w212 _ _ _ _ _ _ _]
          tunnel: w129 -> [_ _ _ w211 _ _ _ _ _ _ _]
          tunnel: w128 -> [_ _ _ w210 _ _ _ _ _ _ _]
          tunnel: w127 -> [_ _ _ _ w237 w334 w431 w528 w625 w722 w819]
          tunnel: w126 -> [_ _ _ _ w236 w333 w430 w527 w624 w721 w818]
          tunnel: w125 -> [_ _ _ _ w232 w329 w426 w523 w620 w717 w814]
          frame 0, Default {
            "Exp 0" <- TRUE
          }
          frame 1 {
            "Exp 2" <- TRUE
          }
          frame 2 {
            # "inital guess\nnormal param with exp 15 and 7.6\nbuzzi ferrari 8.97 and 7.6"
            # "Initial Guesses for the parameters"
            n26 = call <vilib>:"New Session.vi"("Path to Python Module (.py File)"=path "C:/Users/User/Documents/LabVIEW Data/2015 Projects/Combined/WriteTFC.py") -> ("error out"=w179:errorcluster, "Session ID out"=w178:T4)  [unwired: 9 in]
            n27 = call <vilib>:"Pack.vi"("Argument"=w169, "error in (no error)"=w179, "Session ID"=w178) -> ("error out"=w180:errorcluster, "Python Object References Out"=w184:T5, "Session ID out"=w177:T4)  [unwired: 6 in]
            n28 = call <vilib>:"Pack.vi"("Argument"=w168, "error in (no error)"=w180, "Python Object References In"=w184, "Session ID"=w177) -> ("error out"=w181:errorcluster, "Python Object References Out"=w185:T5, "Session ID out"=w187:T4)  [unwired: 5 in]
            n29 = call <vilib>:"Pack.vi"("Argument"=w167, "error in (no error)"=w181, "Python Object References In"=w185, "Session ID"=w187) -> ("error out"=w182:errorcluster, "Python Object References Out"=w186:T5, "Session ID out"=w173:T4)  [unwired: 5 in]
            n30 = call <vilib>:"Pack.vi"("Argument"=w166, "error in (no error)"=w182, "Python Object References In"=w186, "Session ID"=w173) -> ("error out"=w170:errorcluster, "Python Object References Out"=w171:T5, "Session ID out"=w172:T4)  [unwired: 5 in]
            n31 = call <vilib>:"Call.vi"("Function or Method Name"="AppendResultFile", "error in (no error)"=w170, "Python Object References In"=w171, "Session ID"=w172) -> ("error out"=w183:errorcluster, "Session ID out"=w174:T4)  [unwired: 5 in, 1 out]
            n32 = call <vilib>:"Close Session.vi"("error in (no error)"=w183, "Session ID"=w174) -> ()  [unwired: 9 in, 1 out]
            n33 = call <vilib>:"New Session.vi"("Path to Python Module (.py File)"=path "C:/Users/User/Documents/LabVIEW Data/2015 Projects/Combined/initialise.py") -> ("error out"=w159:errorcluster, "Session ID out"=w163:T4)  [unwired: 9 in]
            n34 = call <vilib>:"Pack.vi"("Argument"=8.97, "error in (no error)"=w159, "Session ID"=w163) -> ("error out"=w158:errorcluster, "Python Object References Out"=w156:T5, "Session ID out"=w162:T4)  [unwired: 6 in]
            n35 = call <vilib>:"Pack.vi"("Argument"=7.6, "error in (no error)"=w158, "Python Object References In"=w156, "Session ID"=w162) -> ("error out"=w157:errorcluster, "Python Object References Out"=w155:T5, "Session ID out"=w161:T4)  [unwired: 5 in]
            n36 = call <vilib>:"Call.vi"("Function or Method Name"="initialise", "error in (no error)"=w157, "Python Object References In"=w155, "Session ID"=w161) -> ("error out"=w164:errorcluster, "Session ID out"=w160:T4)  [unwired: 5 in, 1 out]
            n37 = call <vilib>:"Close Session.vi"("error in (no error)"=w164, "Session ID"=w160) -> ()  [unwired: 9 in, 1 out]
            "Temp 1" <- w168
            "Flow 1" <- w167
            "Conc 1" <- w166
            "Exp 1" <- TRUE
          }
          frame 3 {
            n38 = call <vilib>:"New Session.vi"("Path to Python Module (.py File)"=path "C:/Users/User/Documents/LabVIEW Data/2015 Projects/Combined/WriteTFC2ndrow.py") -> ("error out"=w223:errorcluster, "Session ID out"=w222:T4)  [unwired: 9 in]
            n39 = call <vilib>:"Pack.vi"("Argument"=w188, "error in (no error)"=w223, "Session ID"=w222) -> ("error out"=w224:errorcluster, "Python Object References Out"=w228:T5, "Session ID out"=w221:T4)  [unwired: 6 in]
            n40 = call <vilib>:"Pack.vi"("Argument"=w212, "error in (no error)"=w224, "Python Object References In"=w228, "Session ID"=w221) -> ("error out"=w225:errorcluster, "Python Object References Out"=w229:T5, "Session ID out"=w231:T4)  [unwired: 5 in]
            n41 = call <vilib>:"Pack.vi"("Argument"=w211, "error in (no error)"=w225, "Python Object References In"=w229, "Session ID"=w231) -> ("error out"=w226:errorcluster, "Python Object References Out"=w230:T5, "Session ID out"=w217:T4)  [unwired: 5 in]
            n42 = call <vilib>:"Pack.vi"("Argument"=w210, "error in (no error)"=w226, "Python Object References In"=w230, "Session ID"=w217) -> ("error out"=w214:errorcluster, "Python Object References Out"=w215:T5, "Session ID out"=w216:T4)  [unwired: 5 in]
            n43 = call <vilib>:"Call.vi"("Function or Method Name"="AppendResultFile", "error in (no error)"=w214, "Python Object References In"=w215, "Session ID"=w216) -> ("error out"=w227:errorcluster, "Session ID out"=w218:T4)  [unwired: 5 in, 1 out]
            n44 = call <vilib>:"Close Session.vi"("error in (no error)"=w227, "Session ID"=w218) -> ()  [unwired: 9 in, 1 out]
            n45 = call <vilib>:"New Session.vi"("Path to Python Module (.py File)"=path "C:/Users/User/Documents/LabVIEW Data/2015 Projects/Combined/HPLCandAppend.py") -> ("error out"=w206:errorcluster, "Session ID out"=w205:T4)  [unwired: 9 in]
            n46 = call <vilib>:"Pack.vi"("Argument"=w189, "error in (no error)"=w206, "Session ID"=w205) -> ("error out"=w191:errorcluster, "Python Object References Out"=w193:T5, "Session ID out"=w195:T4)  [unwired: 6 in]
            n47 = call <vilib>:"Pack.vi"("Argument"=w188, "error in (no error)"=w191, "Python Object References In"=w193, "Session ID"=w195) -> ("error out"=w190:errorcluster, "Python Object References Out"=w192:T5, "Session ID out"=w194:T4)  [unwired: 5 in]
            n48 = call <vilib>:"Call.vi"("Function or Method Name"="HPLC", "error in (no error)"=w190, "Python Object References In"=w192, "Session ID"=w194) -> ("error out"=w207:errorcluster, "Python Object References Out"=w198:T5, "Session ID out"=w199:T4)  [unwired: 5 in]
            n49 = call-poly <vilib>:"Unpack.vi"("error in (no error)"=w207, "Python Object References In"=w198, "Session ID"=w199) -> ("error out"=w208:errorcluster, "Value"=→"C BAcid 1":dbl, "Python Object References Out"=w203:T5, "Session ID out"=w202:T4)  [unwired: 5 in]
            n50 = call-poly <vilib>:"Unpack.vi"("error in (no error)"=w208, "Python Object References In"=w203, "Session ID"=w202) -> ("error out"=w209:errorcluster, "Value"=→"C EB 1":dbl, "Session ID out"=w204:T4)  [unwired: 5 in, 1 out]
            n51 = call <vilib>:"Close Session.vi"("error in (no error)"=w209, "Session ID"=w204) -> ()  [unwired: 9 in, 1 out]
            "Exp 2" <- TRUE
            "Temp 2" <- w212
            "Flow 2" <- w211
            "Conc 2" <- w210
          }
          frame 4 {
            n52 = flat-sequence {
              tunnel: w240 -> [w248]
              tunnel: w239 -> [w241]
              tunnel: w239 -> [w312]
              tunnel: w237 -> [w292]
              tunnel: w236 -> [w291]
              tunnel: [w275] -> w235
              tunnel: [w274] -> w234
              tunnel: [w273] -> w233
              tunnel: w232 -> [w263]
              frame #0 {
                # "make this include a write to record file step"
                n53 = call <vilib>:"New Session.vi"("Path to Python Module (.py File)"=path "C:/Users/User/Documents/LabVIEW Data/2015 Projects/Combined/HPLCandAppend.py") -> ("error out"=w259:errorcluster, "Session ID out"=w258:T4)  [unwired: 9 in]
                n54 = call <vilib>:"Pack.vi"("Argument"=w248, "error in (no error)"=w259, "Session ID"=w258) -> ("error out"=w243:errorcluster, "Python Object References Out"=w245:T5, "Session ID out"=w247:T4)  [unwired: 6 in]
                n55 = call <vilib>:"Pack.vi"("Argument"=w241, "error in (no error)"=w243, "Python Object References In"=w245, "Session ID"=w247) -> ("error out"=w242:errorcluster, "Python Object References Out"=w244:T5, "Session ID out"=w246:T4)  [unwired: 5 in]
                n56 = call <vilib>:"Call.vi"("Function or Method Name"="HPLC", "error in (no error)"=w242, "Python Object References In"=w244, "Session ID"=w246) -> ("error out"=w260:errorcluster, "Python Object References Out"=w251:T5, "Session ID out"=w252:T4)  [unwired: 5 in]
                n57 = call-poly <vilib>:"Unpack.vi"("error in (no error)"=w260, "Python Object References In"=w251, "Session ID"=w252) -> ("error out"=w261:errorcluster, "Value"=→"C BAcid 2":dbl, "Python Object References Out"=w256:T5, "Session ID out"=w255:T4)  [unwired: 5 in]
                n58 = call-poly <vilib>:"Unpack.vi"("error in (no error)"=w261, "Python Object References In"=w256, "Session ID"=w255) -> ("error out"=w262:errorcluster, "Value"=→"C EB 2":dbl, "Session ID out"=w257:T4)  [unwired: 5 in, 1 out]
                n59 = call <vilib>:"Close Session.vi"("error in (no error)"=w262, "Session ID"=w257) -> ()  [unwired: 9 in, 1 out]
              }
              frame #1 {
                # "Number read"
                n60 = call <vilib>:"New Session.vi"("Path to Python Module (.py File)"=path "C:/Users/User/Documents/LabVIEW Data/2015 Projects/Combined/closed_loop_benzoic_acid.py") -> ("error out"=w317:errorcluster, "Session ID out"=w316:T4)  [unwired: 9 in]
                n61 = call <vilib>:"Pack.vi"("Argument"=w312, "error in (no error)"=w317, "Session ID"=w316) -> ("error out"=w294:errorcluster, "Python Object References Out"=w296:T5, "Session ID out"=w298:T4)  [unwired: 6 in]
                n62 = call <vilib>:"Pack.vi"("Argument"=w292, "error in (no error)"=w294, "Python Object References In"=w296, "Session ID"=w298) -> ("error out"=w293:errorcluster, "Python Object References Out"=w295:T5, "Session ID out"=w297:T4)  [unwired: 5 in]
                n63 = call <vilib>:"Pack.vi"("Argument"=w291, "error in (no error)"=w293, "Python Object References In"=w295, "Session ID"=w297) -> ("error out"=w264:errorcluster, "Python Object References Out"=w267:T5, "Session ID out"=w269:T4)  [unwired: 5 in]
                n64 = call <vilib>:"Pack.vi"("Argument"=w263, "error in (no error)"=w264, "Python Object References In"=w267, "Session ID"=w269) -> ("error out"=w265:errorcluster, "Python Object References Out"=w266:T5, "Session ID out"=w268:T4)  [unwired: 5 in]
                n65 = call <vilib>:"Call.vi"("Function or Method Name"="design_next_experiment", "error in (no error)"=w265, "Python Object References In"=w266, "Session ID"=w268) -> ("error out"=w278:errorcluster, "Python Object References Out"=w281:T5, "Session ID out"=w284:T4)  [unwired: 5 in]
                n66 = call-poly <vilib>:"Unpack.vi"("error in (no error)"=w278, "Python Object References In"=w281, "Session ID"=w284) -> ("error out"=w277:errorcluster, "Value"=w273:dbl, "Python Object References Out"=w280:T5, "Session ID out"=w283:T4)  [unwired: 5 in]
                "Temp 3" <- w273
                n67 = call-poly <vilib>:"Unpack.vi"("error in (no error)"=w277, "Python Object References In"=w280, "Session ID"=w283) -> ("error out"=w276:errorcluster, "Value"=w274:dbl, "Python Object References Out"=w279:T5, "Session ID out"=w282:T4)  [unwired: 5 in]
                "Flow 3" <- w274
                n68 = call-poly <vilib>:"Unpack.vi"("error in (no error)"=w276, "Python Object References In"=w279, "Session ID"=w282) -> ("error out"=w270:errorcluster, "Value"=w275:dbl, "Python Object References Out"=w271:T5, "Session ID out"=w272:T4)  [unwired: 5 in]
                "Conc 3" <- w275
                n69 = call-poly <vilib>:"Unpack.vi"("error in (no error)"=w270, "Python Object References In"=w271, "Session ID"=w272) -> ("error out"=w322:errorcluster, "Value"=→"Param 1 2":dbl, "Python Object References Out"=w320:T5, "Session ID out"=w318:T4)  [unwired: 5 in]
                n70 = call-poly <vilib>:"Unpack.vi"("error in (no error)"=w322, "Python Object References In"=w320, "Session ID"=w318) -> ("error out"=w323:errorcluster, "Value"=→"T value 1 2":dbl, "Python Object References Out"=w321:T5, "Session ID out"=w319:T4)  [unwired: 5 in]
                n71 = call-poly <vilib>:"Unpack.vi"("error in (no error)"=w323, "Python Object References In"=w321, "Session ID"=w319) -> ("error out"=w324:errorcluster, "Value"=→"Param 2 2":dbl, "Python Object References Out"=w315:T5, "Session ID out"=w314:T4)  [unwired: 5 in]
                n72 = call-poly <vilib>:"Unpack.vi"("error in (no error)"=w324, "Python Object References In"=w315, "Session ID"=w314) -> ("error out"=w306:errorcluster, "Value"=→"T value 2 2":dbl, "Python Object References Out"=w308:T5, "Session ID out"=w310:T4)  [unwired: 5 in]
                n73 = call-poly <vilib>:"Unpack.vi"("error in (no error)"=w306, "Python Object References In"=w308, "Session ID"=w310) -> ("error out"=w305:errorcluster, "Value"=→"T Ref 2":dbl, "Python Object References Out"=w307:T5, "Session ID out"=w309:T4)  [unwired: 5 in]
                n74 = call-poly <vilib>:"Unpack.vi"("error in (no error)"=w305, "Python Object References In"=w307, "Session ID"=w309) -> ("error out"=w288:errorcluster, "Value"=→"Correlation 2":dbl, "Python Object References Out"=w289:T5, "Session ID out"=w290:T4)  [unwired: 5 in]
                n75 = call-poly <vilib>:"Unpack.vi"("error in (no error)"=w288, "Python Object References In"=w289, "Session ID"=w290) -> ("error out"=w302:errorcluster, "Value"=→"X2 2":dbl, "Python Object References Out"=w301:T5, "Session ID out"=w300:T4)  [unwired: 5 in]
                n76 = call-poly <vilib>:"Unpack.vi"("error in (no error)"=w302, "Python Object References In"=w301, "Session ID"=w300) -> ("error out"=w285:errorcluster, "Value"=→"X2 ref 2":dbl, "Session ID out"=w286:T4)  [unwired: 5 in, 1 out]
                n77 = call <vilib>:"Close Session.vi"("error in (no error)"=w285, "Session ID"=w286) -> ()  [unwired: 9 in, 1 out]
              }
            }
            "Exp 3" <- TRUE
          }
          frame 5 {
            n78 = flat-sequence {
              tunnel: w337 -> [w345]
              tunnel: w336 -> [w338]
              tunnel: w336 -> [w409]
              tunnel: w334 -> [w389]
              tunnel: w333 -> [w388]
              tunnel: [w372] -> w332
              tunnel: [w371] -> w331
              tunnel: [w370] -> w330
              tunnel: w329 -> [w360]
              frame #0 {
                # "make this include a write to record file step"
                n79 = call <vilib>:"New Session.vi"("Path to Python Module (.py File)"=path "C:/Users/User/Documents/LabVIEW Data/2015 Projects/Combined/HPLCandAppend.py") -> ("error out"=w356:errorcluster, "Session ID out"=w355:T4)  [unwired: 9 in]
                n80 = call <vilib>:"Pack.vi"("Argument"=w345, "error in (no error)"=w356, "Session ID"=w355) -> ("error out"=w340:errorcluster, "Python Object References Out"=w342:T5, "Session ID out"=w344:T4)  [unwired: 6 in]
                n81 = call <vilib>:"Pack.vi"("Argument"=w338, "error in (no error)"=w340, "Python Object References In"=w342, "Session ID"=w344) -> ("error out"=w339:errorcluster, "Python Object References Out"=w341:T5, "Session ID out"=w343:T4)  [unwired: 5 in]
                n82 = call <vilib>:"Call.vi"("Function or Method Name"="HPLC", "error in (no error)"=w339, "Python Object References In"=w341, "Session ID"=w343) -> ("error out"=w357:errorcluster, "Python Object References Out"=w348:T5, "Session ID out"=w349:T4)  [unwired: 5 in]
                n83 = call-poly <vilib>:"Unpack.vi"("error in (no error)"=w357, "Python Object References In"=w348, "Session ID"=w349) -> ("error out"=w358:errorcluster, "Value"=→"C BAcid 3":dbl, "Python Object References Out"=w353:T5, "Session ID out"=w352:T4)  [unwired: 5 in]
                n84 = call-poly <vilib>:"Unpack.vi"("error in (no error)"=w358, "Python Object References In"=w353, "Session ID"=w352) -> ("error out"=w359:errorcluster, "Value"=→"C EB 3":dbl, "Session ID out"=w354:T4)  [unwired: 5 in, 1 out]
                n85 = call <vilib>:"Close Session.vi"("error in (no error)"=w359, "Session ID"=w354) -> ()  [unwired: 9 in, 1 out]
              }
              frame #1 {
                # "Number read"
                n86 = call <vilib>:"New Session.vi"("Path to Python Module (.py File)"=path "C:/Users/User/Documents/LabVIEW Data/2015 Projects/Combined/closed_loop_benzoic_acid.py") -> ("error out"=w414:errorcluster, "Session ID out"=w413:T4)  [unwired: 9 in]
                n87 = call <vilib>:"Pack.vi"("Argument"=w409, "error in (no error)"=w414, "Session ID"=w413) -> ("error out"=w391:errorcluster, "Python Object References Out"=w393:T5, "Session ID out"=w395:T4)  [unwired: 6 in]
                n88 = call <vilib>:"Pack.vi"("Argument"=w389, "error in (no error)"=w391, "Python Object References In"=w393, "Session ID"=w395) -> ("error out"=w390:errorcluster, "Python Object References Out"=w392:T5, "Session ID out"=w394:T4)  [unwired: 5 in]
                n89 = call <vilib>:"Pack.vi"("Argument"=w388, "error in (no error)"=w390, "Python Object References In"=w392, "Session ID"=w394) -> ("error out"=w362:errorcluster, "Python Object References Out"=w364:T5, "Session ID out"=w366:T4)  [unwired: 5 in]
                n90 = call <vilib>:"Pack.vi"("Argument"=w360, "error in (no error)"=w362, "Python Object References In"=w364, "Session ID"=w366) -> ("error out"=w361:errorcluster, "Python Object References Out"=w363:T5, "Session ID out"=w365:T4)  [unwired: 5 in]
                n91 = call <vilib>:"Call.vi"("Function or Method Name"="design_next_experiment", "error in (no error)"=w361, "Python Object References In"=w363, "Session ID"=w365) -> ("error out"=w375:errorcluster, "Python Object References Out"=w378:T5, "Session ID out"=w381:T4)  [unwired: 5 in]
                n92 = call-poly <vilib>:"Unpack.vi"("error in (no error)"=w375, "Python Object References In"=w378, "Session ID"=w381) -> ("error out"=w374:errorcluster, "Value"=w370:dbl, "Python Object References Out"=w377:T5, "Session ID out"=w380:T4)  [unwired: 5 in]
                "Temp 4" <- w370
                n93 = call-poly <vilib>:"Unpack.vi"("error in (no error)"=w374, "Python Object References In"=w377, "Session ID"=w380) -> ("error out"=w373:errorcluster, "Value"=w371:dbl, "Python Object References Out"=w376:T5, "Session ID out"=w379:T4)  [unwired: 5 in]
                "Flow 4" <- w371
                n94 = call-poly <vilib>:"Unpack.vi"("error in (no error)"=w373, "Python Object References In"=w376, "Session ID"=w379) -> ("error out"=w367:errorcluster, "Value"=w372:dbl, "Python Object References Out"=w368:T5, "Session ID out"=w369:T4)  [unwired: 5 in]
                "Conc 4" <- w372
                n95 = call-poly <vilib>:"Unpack.vi"("error in (no error)"=w367, "Python Object References In"=w368, "Session ID"=w369) -> ("error out"=w419:errorcluster, "Value"=→"Param 1 3":dbl, "Python Object References Out"=w417:T5, "Session ID out"=w415:T4)  [unwired: 5 in]
                n96 = call-poly <vilib>:"Unpack.vi"("error in (no error)"=w419, "Python Object References In"=w417, "Session ID"=w415) -> ("error out"=w420:errorcluster, "Value"=→"T value 1 3":dbl, "Python Object References Out"=w418:T5, "Session ID out"=w416:T4)  [unwired: 5 in]
                n97 = call-poly <vilib>:"Unpack.vi"("error in (no error)"=w420, "Python Object References In"=w418, "Session ID"=w416) -> ("error out"=w421:errorcluster, "Value"=→"Param 2 3":dbl, "Python Object References Out"=w412:T5, "Session ID out"=w411:T4)  [unwired: 5 in]
                n98 = call-poly <vilib>:"Unpack.vi"("error in (no error)"=w421, "Python Object References In"=w412, "Session ID"=w411) -> ("error out"=w403:errorcluster, "Value"=→"T value 2 3":dbl, "Python Object References Out"=w405:T5, "Session ID out"=w407:T4)  [unwired: 5 in]
                n99 = call-poly <vilib>:"Unpack.vi"("error in (no error)"=w403, "Python Object References In"=w405, "Session ID"=w407) -> ("error out"=w402:errorcluster, "Value"=→"T Ref 3":dbl, "Python Object References Out"=w404:T5, "Session ID out"=w406:T4)  [unwired: 5 in]
                n100 = call-poly <vilib>:"Unpack.vi"("error in (no error)"=w402, "Python Object References In"=w404, "Session ID"=w406) -> ("error out"=w385:errorcluster, "Value"=→"Correlation 3":dbl, "Python Object References Out"=w386:T5, "Session ID out"=w387:T4)  [unwired: 5 in]
                n101 = call-poly <vilib>:"Unpack.vi"("error in (no error)"=w385, "Python Object References In"=w386, "Session ID"=w387) -> ("error out"=w399:errorcluster, "Value"=→"X2 3":dbl, "Python Object References Out"=w398:T5, "Session ID out"=w397:T4)  [unwired: 5 in]
                n102 = call-poly <vilib>:"Unpack.vi"("error in (no error)"=w399, "Python Object References In"=w398, "Session ID"=w397) -> ("error out"=w382:errorcluster, "Value"=→"X2 ref 3":dbl, "Session ID out"=w383:T4)  [unwired: 5 in, 1 out]
                n103 = call <vilib>:"Close Session.vi"("error in (no error)"=w382, "Session ID"=w383) -> ()  [unwired: 9 in, 1 out]
              }
            }
            "Exp 4" <- TRUE
          }
          frame 6 {
            n104 = flat-sequence {
              tunnel: w434 -> [w442]
              tunnel: w433 -> [w435]
              tunnel: w433 -> [w506]
              tunnel: w431 -> [w486]
              tunnel: w430 -> [w485]
              tunnel: [w469] -> w429
              tunnel: [w468] -> w428
              tunnel: [w467] -> w427
              tunnel: w426 -> [w457]
              frame #0 {
                # "make this include a write to record file step"
                n105 = call <vilib>:"New Session.vi"("Path to Python Module (.py File)"=path "C:/Users/User/Documents/LabVIEW Data/2015 Projects/Combined/HPLCandAppend.py") -> ("error out"=w453:errorcluster, "Session ID out"=w452:T4)  [unwired: 9 in]
                n106 = call <vilib>:"Pack.vi"("Argument"=w442, "error in (no error)"=w453, "Session ID"=w452) -> ("error out"=w437:errorcluster, "Python Object References Out"=w439:T5, "Session ID out"=w441:T4)  [unwired: 6 in]
                n107 = call <vilib>:"Pack.vi"("Argument"=w435, "error in (no error)"=w437, "Python Object References In"=w439, "Session ID"=w441) -> ("error out"=w436:errorcluster, "Python Object References Out"=w438:T5, "Session ID out"=w440:T4)  [unwired: 5 in]
                n108 = call <vilib>:"Call.vi"("Function or Method Name"="HPLC", "error in (no error)"=w436, "Python Object References In"=w438, "Session ID"=w440) -> ("error out"=w454:errorcluster, "Python Object References Out"=w445:T5, "Session ID out"=w446:T4)  [unwired: 5 in]
                n109 = call-poly <vilib>:"Unpack.vi"("error in (no error)"=w454, "Python Object References In"=w445, "Session ID"=w446) -> ("error out"=w455:errorcluster, "Value"=→"C BAcid 4":dbl, "Python Object References Out"=w450:T5, "Session ID out"=w449:T4)  [unwired: 5 in]
                n110 = call-poly <vilib>:"Unpack.vi"("error in (no error)"=w455, "Python Object References In"=w450, "Session ID"=w449) -> ("error out"=w456:errorcluster, "Value"=→"C EB 4":dbl, "Session ID out"=w451:T4)  [unwired: 5 in, 1 out]
                n111 = call <vilib>:"Close Session.vi"("error in (no error)"=w456, "Session ID"=w451) -> ()  [unwired: 9 in, 1 out]
              }
              frame #1 {
                # "Number read"
                n112 = call <vilib>:"New Session.vi"("Path to Python Module (.py File)"=path "C:/Users/User/Documents/LabVIEW Data/2015 Projects/Combined/closed_loop_benzoic_acid.py") -> ("error out"=w511:errorcluster, "Session ID out"=w510:T4)  [unwired: 9 in]
                n113 = call <vilib>:"Pack.vi"("Argument"=w506, "error in (no error)"=w511, "Session ID"=w510) -> ("error out"=w488:errorcluster, "Python Object References Out"=w490:T5, "Session ID out"=w492:T4)  [unwired: 6 in]
                n114 = call <vilib>:"Pack.vi"("Argument"=w486, "error in (no error)"=w488, "Python Object References In"=w490, "Session ID"=w492) -> ("error out"=w487:errorcluster, "Python Object References Out"=w489:T5, "Session ID out"=w491:T4)  [unwired: 5 in]
                n115 = call <vilib>:"Pack.vi"("Argument"=w485, "error in (no error)"=w487, "Python Object References In"=w489, "Session ID"=w491) -> ("error out"=w459:errorcluster, "Python Object References Out"=w460:T5, "Session ID out"=w463:T4)  [unwired: 5 in]
                n116 = call <vilib>:"Pack.vi"("Argument"=w457, "error in (no error)"=w459, "Python Object References In"=w460, "Session ID"=w463) -> ("error out"=w458:errorcluster, "Python Object References Out"=w461:T5, "Session ID out"=w462:T4)  [unwired: 5 in]
                n117 = call <vilib>:"Call.vi"("Function or Method Name"="design_next_experiment", "error in (no error)"=w458, "Python Object References In"=w461, "Session ID"=w462) -> ("error out"=w472:errorcluster, "Python Object References Out"=w475:T5, "Session ID out"=w478:T4)  [unwired: 5 in]
                n118 = call-poly <vilib>:"Unpack.vi"("error in (no error)"=w472, "Python Object References In"=w475, "Session ID"=w478) -> ("error out"=w471:errorcluster, "Value"=w467:dbl, "Python Object References Out"=w474:T5, "Session ID out"=w477:T4)  [unwired: 5 in]
                "Temp 5" <- w467
                n119 = call-poly <vilib>:"Unpack.vi"("error in (no error)"=w471, "Python Object References In"=w474, "Session ID"=w477) -> ("error out"=w470:errorcluster, "Value"=w468:dbl, "Python Object References Out"=w473:T5, "Session ID out"=w476:T4)  [unwired: 5 in]
                "Flow 5" <- w468
                n120 = call-poly <vilib>:"Unpack.vi"("error in (no error)"=w470, "Python Object References In"=w473, "Session ID"=w476) -> ("error out"=w464:errorcluster, "Value"=w469:dbl, "Python Object References Out"=w465:T5, "Session ID out"=w466:T4)  [unwired: 5 in]
                "Conc 5" <- w469
                n121 = call-poly <vilib>:"Unpack.vi"("error in (no error)"=w464, "Python Object References In"=w465, "Session ID"=w466) -> ("error out"=w516:errorcluster, "Value"=→"Param 1 4":dbl, "Python Object References Out"=w514:T5, "Session ID out"=w512:T4)  [unwired: 5 in]
                n122 = call-poly <vilib>:"Unpack.vi"("error in (no error)"=w516, "Python Object References In"=w514, "Session ID"=w512) -> ("error out"=w517:errorcluster, "Value"=→"T value 1 4":dbl, "Python Object References Out"=w515:T5, "Session ID out"=w513:T4)  [unwired: 5 in]
                n123 = call-poly <vilib>:"Unpack.vi"("error in (no error)"=w517, "Python Object References In"=w515, "Session ID"=w513) -> ("error out"=w518:errorcluster, "Value"=→"Param 2 4":dbl, "Python Object References Out"=w509:T5, "Session ID out"=w508:T4)  [unwired: 5 in]
                n124 = call-poly <vilib>:"Unpack.vi"("error in (no error)"=w518, "Python Object References In"=w509, "Session ID"=w508) -> ("error out"=w500:errorcluster, "Value"=→"T value 2 4":dbl, "Python Object References Out"=w502:T5, "Session ID out"=w504:T4)  [unwired: 5 in]
                n125 = call-poly <vilib>:"Unpack.vi"("error in (no error)"=w500, "Python Object References In"=w502, "Session ID"=w504) -> ("error out"=w499:errorcluster, "Value"=→"T Ref 4":dbl, "Python Object References Out"=w501:T5, "Session ID out"=w503:T4)  [unwired: 5 in]
                n126 = call-poly <vilib>:"Unpack.vi"("error in (no error)"=w499, "Python Object References In"=w501, "Session ID"=w503) -> ("error out"=w482:errorcluster, "Value"=→"Correlation 4":dbl, "Python Object References Out"=w483:T5, "Session ID out"=w484:T4)  [unwired: 5 in]
                n127 = call-poly <vilib>:"Unpack.vi"("error in (no error)"=w482, "Python Object References In"=w483, "Session ID"=w484) -> ("error out"=w496:errorcluster, "Value"=→"X2 4":dbl, "Python Object References Out"=w495:T5, "Session ID out"=w494:T4)  [unwired: 5 in]
                n128 = call-poly <vilib>:"Unpack.vi"("error in (no error)"=w496, "Python Object References In"=w495, "Session ID"=w494) -> ("error out"=w479:errorcluster, "Value"=→"X2 ref 4":dbl, "Session ID out"=w480:T4)  [unwired: 5 in, 1 out]
                n129 = call <vilib>:"Close Session.vi"("error in (no error)"=w479, "Session ID"=w480) -> ()  [unwired: 9 in, 1 out]
              }
            }
            "Exp 5" <- TRUE
          }
          frame 7 {
            n130 = flat-sequence {
              tunnel: w531 -> [w539]
              tunnel: w530 -> [w532]
              tunnel: w530 -> [w603]
              tunnel: w528 -> [w583]
              tunnel: w527 -> [w582]
              tunnel: [w566] -> w526
              tunnel: [w565] -> w525
              tunnel: [w564] -> w524
              tunnel: w523 -> [w554]
              frame #0 {
                # "make this include a write to record file step"
                n131 = call <vilib>:"New Session.vi"("Path to Python Module (.py File)"=path "C:/Users/User/Documents/LabVIEW Data/2015 Projects/Combined/HPLCandAppend.py") -> ("error out"=w550:errorcluster, "Session ID out"=w549:T4)  [unwired: 9 in]
                n132 = call <vilib>:"Pack.vi"("Argument"=w539, "error in (no error)"=w550, "Session ID"=w549) -> ("error out"=w534:errorcluster, "Python Object References Out"=w536:T5, "Session ID out"=w538:T4)  [unwired: 6 in]
                n133 = call <vilib>:"Pack.vi"("Argument"=w532, "error in (no error)"=w534, "Python Object References In"=w536, "Session ID"=w538) -> ("error out"=w533:errorcluster, "Python Object References Out"=w535:T5, "Session ID out"=w537:T4)  [unwired: 5 in]
                n134 = call <vilib>:"Call.vi"("Function or Method Name"="HPLC", "error in (no error)"=w533, "Python Object References In"=w535, "Session ID"=w537) -> ("error out"=w551:errorcluster, "Python Object References Out"=w542:T5, "Session ID out"=w543:T4)  [unwired: 5 in]
                n135 = call-poly <vilib>:"Unpack.vi"("error in (no error)"=w551, "Python Object References In"=w542, "Session ID"=w543) -> ("error out"=w552:errorcluster, "Value"=→"C BAcid 5":dbl, "Python Object References Out"=w547:T5, "Session ID out"=w546:T4)  [unwired: 5 in]
                n136 = call-poly <vilib>:"Unpack.vi"("error in (no error)"=w552, "Python Object References In"=w547, "Session ID"=w546) -> ("error out"=w553:errorcluster, "Value"=→"C EB 5":dbl, "Session ID out"=w548:T4)  [unwired: 5 in, 1 out]
                n137 = call <vilib>:"Close Session.vi"("error in (no error)"=w553, "Session ID"=w548) -> ()  [unwired: 9 in, 1 out]
              }
              frame #1 {
                # "Number read"
                n138 = call <vilib>:"New Session.vi"("Path to Python Module (.py File)"=path "C:/Users/User/Documents/LabVIEW Data/2015 Projects/Combined/closed_loop_benzoic_acid.py") -> ("error out"=w608:errorcluster, "Session ID out"=w607:T4)  [unwired: 9 in]
                n139 = call <vilib>:"Pack.vi"("Argument"=w603, "error in (no error)"=w608, "Session ID"=w607) -> ("error out"=w585:errorcluster, "Python Object References Out"=w587:T5, "Session ID out"=w589:T4)  [unwired: 6 in]
                n140 = call <vilib>:"Pack.vi"("Argument"=w583, "error in (no error)"=w585, "Python Object References In"=w587, "Session ID"=w589) -> ("error out"=w584:errorcluster, "Python Object References Out"=w586:T5, "Session ID out"=w588:T4)  [unwired: 5 in]
                n141 = call <vilib>:"Pack.vi"("Argument"=w582, "error in (no error)"=w584, "Python Object References In"=w586, "Session ID"=w588) -> ("error out"=w555:errorcluster, "Python Object References Out"=w558:T5, "Session ID out"=w560:T4)  [unwired: 5 in]
                n142 = call <vilib>:"Pack.vi"("Argument"=w554, "error in (no error)"=w555, "Python Object References In"=w558, "Session ID"=w560) -> ("error out"=w556:errorcluster, "Python Object References Out"=w557:T5, "Session ID out"=w559:T4)  [unwired: 5 in]
                n143 = call <vilib>:"Call.vi"("Function or Method Name"="design_next_experiment", "error in (no error)"=w556, "Python Object References In"=w557, "Session ID"=w559) -> ("error out"=w569:errorcluster, "Python Object References Out"=w572:T5, "Session ID out"=w575:T4)  [unwired: 5 in]
                n144 = call-poly <vilib>:"Unpack.vi"("error in (no error)"=w569, "Python Object References In"=w572, "Session ID"=w575) -> ("error out"=w568:errorcluster, "Value"=w564:dbl, "Python Object References Out"=w571:T5, "Session ID out"=w574:T4)  [unwired: 5 in]
                "Temp 6" <- w564
                n145 = call-poly <vilib>:"Unpack.vi"("error in (no error)"=w568, "Python Object References In"=w571, "Session ID"=w574) -> ("error out"=w567:errorcluster, "Value"=w565:dbl, "Python Object References Out"=w570:T5, "Session ID out"=w573:T4)  [unwired: 5 in]
                "Flow 6" <- w565
                n146 = call-poly <vilib>:"Unpack.vi"("error in (no error)"=w567, "Python Object References In"=w570, "Session ID"=w573) -> ("error out"=w561:errorcluster, "Value"=w566:dbl, "Python Object References Out"=w562:T5, "Session ID out"=w563:T4)  [unwired: 5 in]
                "Conc 6" <- w566
                n147 = call-poly <vilib>:"Unpack.vi"("error in (no error)"=w561, "Python Object References In"=w562, "Session ID"=w563) -> ("error out"=w613:errorcluster, "Value"=→"Param 1 5":dbl, "Python Object References Out"=w611:T5, "Session ID out"=w609:T4)  [unwired: 5 in]
                n148 = call-poly <vilib>:"Unpack.vi"("error in (no error)"=w613, "Python Object References In"=w611, "Session ID"=w609) -> ("error out"=w614:errorcluster, "Value"=→"T value 1 5":dbl, "Python Object References Out"=w612:T5, "Session ID out"=w610:T4)  [unwired: 5 in]
                n149 = call-poly <vilib>:"Unpack.vi"("error in (no error)"=w614, "Python Object References In"=w612, "Session ID"=w610) -> ("error out"=w615:errorcluster, "Value"=→"Param 2 5":dbl, "Python Object References Out"=w606:T5, "Session ID out"=w605:T4)  [unwired: 5 in]
                n150 = call-poly <vilib>:"Unpack.vi"("error in (no error)"=w615, "Python Object References In"=w606, "Session ID"=w605) -> ("error out"=w597:errorcluster, "Value"=→"T value 2 5":dbl, "Python Object References Out"=w599:T5, "Session ID out"=w601:T4)  [unwired: 5 in]
                n151 = call-poly <vilib>:"Unpack.vi"("error in (no error)"=w597, "Python Object References In"=w599, "Session ID"=w601) -> ("error out"=w596:errorcluster, "Value"=→"T Ref 5":dbl, "Python Object References Out"=w598:T5, "Session ID out"=w600:T4)  [unwired: 5 in]
                n152 = call-poly <vilib>:"Unpack.vi"("error in (no error)"=w596, "Python Object References In"=w598, "Session ID"=w600) -> ("error out"=w579:errorcluster, "Value"=→"Correlation 5":dbl, "Python Object References Out"=w580:T5, "Session ID out"=w581:T4)  [unwired: 5 in]
                n153 = call-poly <vilib>:"Unpack.vi"("error in (no error)"=w579, "Python Object References In"=w580, "Session ID"=w581) -> ("error out"=w593:errorcluster, "Value"=→"X2 5":dbl, "Python Object References Out"=w592:T5, "Session ID out"=w591:T4)  [unwired: 5 in]
                n154 = call-poly <vilib>:"Unpack.vi"("error in (no error)"=w593, "Python Object References In"=w592, "Session ID"=w591) -> ("error out"=w576:errorcluster, "Value"=→"X2 ref 5":dbl, "Session ID out"=w577:T4)  [unwired: 5 in, 1 out]
                n155 = call <vilib>:"Close Session.vi"("error in (no error)"=w576, "Session ID"=w577) -> ()  [unwired: 9 in, 1 out]
              }
            }
            "Exp 6" <- TRUE
          }
          frame 8 {
            n156 = flat-sequence {
              tunnel: w628 -> [w636]
              tunnel: w627 -> [w629]
              tunnel: w627 -> [w700]
              tunnel: w625 -> [w680]
              tunnel: w624 -> [w679]
              tunnel: [w663] -> w623
              tunnel: [w662] -> w622
              tunnel: [w661] -> w621
              tunnel: w620 -> [w651]
              frame #0 {
                # "make this include a write to record file step"
                n157 = call <vilib>:"New Session.vi"("Path to Python Module (.py File)"=path "C:/Users/User/Documents/LabVIEW Data/2015 Projects/Combined/HPLCandAppend.py") -> ("error out"=w647:errorcluster, "Session ID out"=w646:T4)  [unwired: 9 in]
                n158 = call <vilib>:"Pack.vi"("Argument"=w636, "error in (no error)"=w647, "Session ID"=w646) -> ("error out"=w631:errorcluster, "Python Object References Out"=w633:T5, "Session ID out"=w635:T4)  [unwired: 6 in]
                n159 = call <vilib>:"Pack.vi"("Argument"=w629, "error in (no error)"=w631, "Python Object References In"=w633, "Session ID"=w635) -> ("error out"=w630:errorcluster, "Python Object References Out"=w632:T5, "Session ID out"=w634:T4)  [unwired: 5 in]
                n160 = call <vilib>:"Call.vi"("Function or Method Name"="HPLC", "error in (no error)"=w630, "Python Object References In"=w632, "Session ID"=w634) -> ("error out"=w648:errorcluster, "Python Object References Out"=w639:T5, "Session ID out"=w640:T4)  [unwired: 5 in]
                n161 = call-poly <vilib>:"Unpack.vi"("error in (no error)"=w648, "Python Object References In"=w639, "Session ID"=w640) -> ("error out"=w649:errorcluster, "Value"=→"C BAcid 6":dbl, "Python Object References Out"=w644:T5, "Session ID out"=w643:T4)  [unwired: 5 in]
                n162 = call-poly <vilib>:"Unpack.vi"("error in (no error)"=w649, "Python Object References In"=w644, "Session ID"=w643) -> ("error out"=w650:errorcluster, "Value"=→"C EB 6":dbl, "Session ID out"=w645:T4)  [unwired: 5 in, 1 out]
                n163 = call <vilib>:"Close Session.vi"("error in (no error)"=w650, "Session ID"=w645) -> ()  [unwired: 9 in, 1 out]
              }
              frame #1 {
                # "Number read"
                n164 = call <vilib>:"New Session.vi"("Path to Python Module (.py File)"=path "C:/Users/User/Documents/LabVIEW Data/2015 Projects/Combined/closed_loop_benzoic_acid.py") -> ("error out"=w705:errorcluster, "Session ID out"=w704:T4)  [unwired: 9 in]
                n165 = call <vilib>:"Pack.vi"("Argument"=w700, "error in (no error)"=w705, "Session ID"=w704) -> ("error out"=w682:errorcluster, "Python Object References Out"=w684:T5, "Session ID out"=w686:T4)  [unwired: 6 in]
                n166 = call <vilib>:"Pack.vi"("Argument"=w680, "error in (no error)"=w682, "Python Object References In"=w684, "Session ID"=w686) -> ("error out"=w681:errorcluster, "Python Object References Out"=w683:T5, "Session ID out"=w685:T4)  [unwired: 5 in]
                n167 = call <vilib>:"Pack.vi"("Argument"=w679, "error in (no error)"=w681, "Python Object References In"=w683, "Session ID"=w685) -> ("error out"=w652:errorcluster, "Python Object References Out"=w655:T5, "Session ID out"=w657:T4)  [unwired: 5 in]
                n168 = call <vilib>:"Pack.vi"("Argument"=w651, "error in (no error)"=w652, "Python Object References In"=w655, "Session ID"=w657) -> ("error out"=w653:errorcluster, "Python Object References Out"=w654:T5, "Session ID out"=w656:T4)  [unwired: 5 in]
                n169 = call <vilib>:"Call.vi"("Function or Method Name"="design_next_experiment", "error in (no error)"=w653, "Python Object References In"=w654, "Session ID"=w656) -> ("error out"=w666:errorcluster, "Python Object References Out"=w669:T5, "Session ID out"=w672:T4)  [unwired: 5 in]
                n170 = call-poly <vilib>:"Unpack.vi"("error in (no error)"=w666, "Python Object References In"=w669, "Session ID"=w672) -> ("error out"=w665:errorcluster, "Value"=w661:dbl, "Python Object References Out"=w668:T5, "Session ID out"=w671:T4)  [unwired: 5 in]
                "Temp 7" <- w661
                n171 = call-poly <vilib>:"Unpack.vi"("error in (no error)"=w665, "Python Object References In"=w668, "Session ID"=w671) -> ("error out"=w664:errorcluster, "Value"=w662:dbl, "Python Object References Out"=w667:T5, "Session ID out"=w670:T4)  [unwired: 5 in]
                "Flow 7" <- w662
                n172 = call-poly <vilib>:"Unpack.vi"("error in (no error)"=w664, "Python Object References In"=w667, "Session ID"=w670) -> ("error out"=w658:errorcluster, "Value"=w663:dbl, "Python Object References Out"=w659:T5, "Session ID out"=w660:T4)  [unwired: 5 in]
                "Conc 7" <- w663
                n173 = call-poly <vilib>:"Unpack.vi"("error in (no error)"=w658, "Python Object References In"=w659, "Session ID"=w660) -> ("error out"=w710:errorcluster, "Value"=→"Param 1 6":dbl, "Python Object References Out"=w708:T5, "Session ID out"=w706:T4)  [unwired: 5 in]
                n174 = call-poly <vilib>:"Unpack.vi"("error in (no error)"=w710, "Python Object References In"=w708, "Session ID"=w706) -> ("error out"=w711:errorcluster, "Value"=→"T value 1 6":dbl, "Python Object References Out"=w709:T5, "Session ID out"=w707:T4)  [unwired: 5 in]
                n175 = call-poly <vilib>:"Unpack.vi"("error in (no error)"=w711, "Python Object References In"=w709, "Session ID"=w707) -> ("error out"=w712:errorcluster, "Value"=→"Param 2 6":dbl, "Python Object References Out"=w703:T5, "Session ID out"=w702:T4)  [unwired: 5 in]
                n176 = call-poly <vilib>:"Unpack.vi"("error in (no error)"=w712, "Python Object References In"=w703, "Session ID"=w702) -> ("error out"=w694:errorcluster, "Value"=→"T value 2 6":dbl, "Python Object References Out"=w696:T5, "Session ID out"=w698:T4)  [unwired: 5 in]
                n177 = call-poly <vilib>:"Unpack.vi"("error in (no error)"=w694, "Python Object References In"=w696, "Session ID"=w698) -> ("error out"=w693:errorcluster, "Value"=→"T Ref 6":dbl, "Python Object References Out"=w695:T5, "Session ID out"=w697:T4)  [unwired: 5 in]
                n178 = call-poly <vilib>:"Unpack.vi"("error in (no error)"=w693, "Python Object References In"=w695, "Session ID"=w697) -> ("error out"=w676:errorcluster, "Value"=→"Correlation 6":dbl, "Python Object References Out"=w677:T5, "Session ID out"=w678:T4)  [unwired: 5 in]
                n179 = call-poly <vilib>:"Unpack.vi"("error in (no error)"=w676, "Python Object References In"=w677, "Session ID"=w678) -> ("error out"=w690:errorcluster, "Value"=→"X2 6":dbl, "Python Object References Out"=w689:T5, "Session ID out"=w688:T4)  [unwired: 5 in]
                n180 = call-poly <vilib>:"Unpack.vi"("error in (no error)"=w690, "Python Object References In"=w689, "Session ID"=w688) -> ("error out"=w673:errorcluster, "Value"=→"X2 ref 6":dbl, "Session ID out"=w674:T4)  [unwired: 5 in, 1 out]
                n181 = call <vilib>:"Close Session.vi"("error in (no error)"=w673, "Session ID"=w674) -> ()  [unwired: 9 in, 1 out]
              }
            }
            "Exp 7" <- TRUE
          }
          frame 9 {
            n182 = flat-sequence {
              tunnel: w725 -> [w733]
              tunnel: w724 -> [w726]
              tunnel: w724 -> [w797]
              tunnel: w722 -> [w777]
              tunnel: w721 -> [w776]
              tunnel: [w760] -> w720
              tunnel: [w759] -> w719
              tunnel: [w758] -> w718
              tunnel: w717 -> [w748]
              frame #0 {
                # "make this include a write to record file step"
                n183 = call <vilib>:"New Session.vi"("Path to Python Module (.py File)"=path "C:/Users/User/Documents/LabVIEW Data/2015 Projects/Combined/HPLCandAppend.py") -> ("error out"=w744:errorcluster, "Session ID out"=w743:T4)  [unwired: 9 in]
                n184 = call <vilib>:"Pack.vi"("Argument"=w733, "error in (no error)"=w744, "Session ID"=w743) -> ("error out"=w728:errorcluster, "Python Object References Out"=w730:T5, "Session ID out"=w732:T4)  [unwired: 6 in]
                n185 = call <vilib>:"Pack.vi"("Argument"=w726, "error in (no error)"=w728, "Python Object References In"=w730, "Session ID"=w732) -> ("error out"=w727:errorcluster, "Python Object References Out"=w729:T5, "Session ID out"=w731:T4)  [unwired: 5 in]
                n186 = call <vilib>:"Call.vi"("Function or Method Name"="HPLC", "error in (no error)"=w727, "Python Object References In"=w729, "Session ID"=w731) -> ("error out"=w745:errorcluster, "Python Object References Out"=w736:T5, "Session ID out"=w737:T4)  [unwired: 5 in]
                n187 = call-poly <vilib>:"Unpack.vi"("error in (no error)"=w745, "Python Object References In"=w736, "Session ID"=w737) -> ("error out"=w746:errorcluster, "Value"=→"C BAcid 7":dbl, "Python Object References Out"=w741:T5, "Session ID out"=w740:T4)  [unwired: 5 in]
                n188 = call-poly <vilib>:"Unpack.vi"("error in (no error)"=w746, "Python Object References In"=w741, "Session ID"=w740) -> ("error out"=w747:errorcluster, "Value"=→"C EB 7":dbl, "Session ID out"=w742:T4)  [unwired: 5 in, 1 out]
                n189 = call <vilib>:"Close Session.vi"("error in (no error)"=w747, "Session ID"=w742) -> ()  [unwired: 9 in, 1 out]
              }
              frame #1 {
                # "Number read"
                n190 = call <vilib>:"New Session.vi"("Path to Python Module (.py File)"=path "C:/Users/User/Documents/LabVIEW Data/2015 Projects/Combined/closed_loop_benzoic_acid.py") -> ("error out"=w802:errorcluster, "Session ID out"=w801:T4)  [unwired: 9 in]
                n191 = call <vilib>:"Pack.vi"("Argument"=w797, "error in (no error)"=w802, "Session ID"=w801) -> ("error out"=w779:errorcluster, "Python Object References Out"=w781:T5, "Session ID out"=w783:T4)  [unwired: 6 in]
                n192 = call <vilib>:"Pack.vi"("Argument"=w777, "error in (no error)"=w779, "Python Object References In"=w781, "Session ID"=w783) -> ("error out"=w778:errorcluster, "Python Object References Out"=w780:T5, "Session ID out"=w782:T4)  [unwired: 5 in]
                n193 = call <vilib>:"Pack.vi"("Argument"=w776, "error in (no error)"=w778, "Python Object References In"=w780, "Session ID"=w782) -> ("error out"=w750:errorcluster, "Python Object References Out"=w752:T5, "Session ID out"=w754:T4)  [unwired: 5 in]
                n194 = call <vilib>:"Pack.vi"("Argument"=w748, "error in (no error)"=w750, "Python Object References In"=w752, "Session ID"=w754) -> ("error out"=w749:errorcluster, "Python Object References Out"=w751:T5, "Session ID out"=w753:T4)  [unwired: 5 in]
                n195 = call <vilib>:"Call.vi"("Function or Method Name"="design_next_experiment", "error in (no error)"=w749, "Python Object References In"=w751, "Session ID"=w753) -> ("error out"=w763:errorcluster, "Python Object References Out"=w766:T5, "Session ID out"=w769:T4)  [unwired: 5 in]
                n196 = call-poly <vilib>:"Unpack.vi"("error in (no error)"=w763, "Python Object References In"=w766, "Session ID"=w769) -> ("error out"=w762:errorcluster, "Value"=w758:dbl, "Python Object References Out"=w765:T5, "Session ID out"=w768:T4)  [unwired: 5 in]
                "Temp 8" <- w758
                n197 = call-poly <vilib>:"Unpack.vi"("error in (no error)"=w762, "Python Object References In"=w765, "Session ID"=w768) -> ("error out"=w761:errorcluster, "Value"=w759:dbl, "Python Object References Out"=w764:T5, "Session ID out"=w767:T4)  [unwired: 5 in]
                "Flow 8" <- w759
                n198 = call-poly <vilib>:"Unpack.vi"("error in (no error)"=w761, "Python Object References In"=w764, "Session ID"=w767) -> ("error out"=w755:errorcluster, "Value"=w760:dbl, "Python Object References Out"=w756:T5, "Session ID out"=w757:T4)  [unwired: 5 in]
                "Conc 8" <- w760
                n199 = call-poly <vilib>:"Unpack.vi"("error in (no error)"=w755, "Python Object References In"=w756, "Session ID"=w757) -> ("error out"=w807:errorcluster, "Value"=→"Param 1 7":dbl, "Python Object References Out"=w805:T5, "Session ID out"=w803:T4)  [unwired: 5 in]
                n200 = call-poly <vilib>:"Unpack.vi"("error in (no error)"=w807, "Python Object References In"=w805, "Session ID"=w803) -> ("error out"=w808:errorcluster, "Value"=→"T value 1 7":dbl, "Python Object References Out"=w806:T5, "Session ID out"=w804:T4)  [unwired: 5 in]
                n201 = call-poly <vilib>:"Unpack.vi"("error in (no error)"=w808, "Python Object References In"=w806, "Session ID"=w804) -> ("error out"=w809:errorcluster, "Value"=→"Param 2 7":dbl, "Python Object References Out"=w800:T5, "Session ID out"=w799:T4)  [unwired: 5 in]
                n202 = call-poly <vilib>:"Unpack.vi"("error in (no error)"=w809, "Python Object References In"=w800, "Session ID"=w799) -> ("error out"=w791:errorcluster, "Value"=→"T value 2 7":dbl, "Python Object References Out"=w793:T5, "Session ID out"=w795:T4)  [unwired: 5 in]
                n203 = call-poly <vilib>:"Unpack.vi"("error in (no error)"=w791, "Python Object References In"=w793, "Session ID"=w795) -> ("error out"=w790:errorcluster, "Value"=→"T Ref 7":dbl, "Python Object References Out"=w792:T5, "Session ID out"=w794:T4)  [unwired: 5 in]
                n204 = call-poly <vilib>:"Unpack.vi"("error in (no error)"=w790, "Python Object References In"=w792, "Session ID"=w794) -> ("error out"=w773:errorcluster, "Value"=→"Correlation 7":dbl, "Python Object References Out"=w774:T5, "Session ID out"=w775:T4)  [unwired: 5 in]
                n205 = call-poly <vilib>:"Unpack.vi"("error in (no error)"=w773, "Python Object References In"=w774, "Session ID"=w775) -> ("error out"=w787:errorcluster, "Value"=→"X2 7":dbl, "Python Object References Out"=w786:T5, "Session ID out"=w785:T4)  [unwired: 5 in]
                n206 = call-poly <vilib>:"Unpack.vi"("error in (no error)"=w787, "Python Object References In"=w786, "Session ID"=w785) -> ("error out"=w770:errorcluster, "Value"=→"X2 ref 7":dbl, "Session ID out"=w771:T4)  [unwired: 5 in, 1 out]
                n207 = call <vilib>:"Close Session.vi"("error in (no error)"=w770, "Session ID"=w771) -> ()  [unwired: 9 in, 1 out]
              }
            }
            "Exp 8" <- TRUE
          }
          frame 10 {
            n208 = flat-sequence {
              tunnel: w822 -> [w830]
              tunnel: w821 -> [w823]
              tunnel: w821 -> [w894]
              tunnel: w819 -> [w874]
              tunnel: w818 -> [w873]
              tunnel: w814 -> [w845]
              frame #0 {
                # "make this include a write to record file step"
                n209 = call <vilib>:"New Session.vi"("Path to Python Module (.py File)"=path "C:/Users/User/Documents/LabVIEW Data/2015 Projects/Combined/HPLCandAppend.py") -> ("error out"=w841:errorcluster, "Session ID out"=w840:T4)  [unwired: 9 in]
                n210 = call <vilib>:"Pack.vi"("Argument"=w830, "error in (no error)"=w841, "Session ID"=w840) -> ("error out"=w825:errorcluster, "Python Object References Out"=w827:T5, "Session ID out"=w829:T4)  [unwired: 6 in]
                n211 = call <vilib>:"Pack.vi"("Argument"=w823, "error in (no error)"=w825, "Python Object References In"=w827, "Session ID"=w829) -> ("error out"=w824:errorcluster, "Python Object References Out"=w826:T5, "Session ID out"=w828:T4)  [unwired: 5 in]
                n212 = call <vilib>:"Call.vi"("Function or Method Name"="HPLC", "error in (no error)"=w824, "Python Object References In"=w826, "Session ID"=w828) -> ("error out"=w842:errorcluster, "Python Object References Out"=w833:T5, "Session ID out"=w834:T4)  [unwired: 5 in]
                n213 = call-poly <vilib>:"Unpack.vi"("error in (no error)"=w842, "Python Object References In"=w833, "Session ID"=w834) -> ("error out"=w843:errorcluster, "Value"=→"C BAcid 8":dbl, "Python Object References Out"=w838:T5, "Session ID out"=w837:T4)  [unwired: 5 in]
                n214 = call-poly <vilib>:"Unpack.vi"("error in (no error)"=w843, "Python Object References In"=w838, "Session ID"=w837) -> ("error out"=w844:errorcluster, "Value"=→"C EB 8":dbl, "Session ID out"=w839:T4)  [unwired: 5 in, 1 out]
                n215 = call <vilib>:"Close Session.vi"("error in (no error)"=w844, "Session ID"=w839) -> ()  [unwired: 9 in, 1 out]
              }
              frame #1 {
                # "Number read"
                n216 = call <vilib>:"New Session.vi"("Path to Python Module (.py File)"=path "C:/Users/User/Documents/LabVIEW Data/2015 Projects/Combined/closed_loop_benzoic_acid.py") -> ("error out"=w899:errorcluster, "Session ID out"=w898:T4)  [unwired: 9 in]
                n217 = call <vilib>:"Pack.vi"("Argument"=w894, "error in (no error)"=w899, "Session ID"=w898) -> ("error out"=w876:errorcluster, "Python Object References Out"=w878:T5, "Session ID out"=w880:T4)  [unwired: 6 in]
                n218 = call <vilib>:"Pack.vi"("Argument"=w874, "error in (no error)"=w876, "Python Object References In"=w878, "Session ID"=w880) -> ("error out"=w875:errorcluster, "Python Object References Out"=w877:T5, "Session ID out"=w879:T4)  [unwired: 5 in]
                n219 = call <vilib>:"Pack.vi"("Argument"=w873, "error in (no error)"=w875, "Python Object References In"=w877, "Session ID"=w879) -> ("error out"=w847:errorcluster, "Python Object References Out"=w849:T5, "Session ID out"=w851:T4)  [unwired: 5 in]
                n220 = call <vilib>:"Pack.vi"("Argument"=w845, "error in (no error)"=w847, "Python Object References In"=w849, "Session ID"=w851) -> ("error out"=w846:errorcluster, "Python Object References Out"=w848:T5, "Session ID out"=w850:T4)  [unwired: 5 in]
                n221 = call <vilib>:"Call.vi"("Function or Method Name"="design_next_experiment", "error in (no error)"=w846, "Python Object References In"=w848, "Session ID"=w850) -> ("error out"=w860:errorcluster, "Python Object References Out"=w863:T5, "Session ID out"=w866:T4)  [unwired: 5 in]
                n222 = call-poly <vilib>:"Unpack.vi"("error in (no error)"=w860, "Python Object References In"=w863, "Session ID"=w866) -> ("error out"=w859:errorcluster, "Value"=→"Temp 9":dbl, "Python Object References Out"=w862:T5, "Session ID out"=w865:T4)  [unwired: 5 in]
                n223 = call-poly <vilib>:"Unpack.vi"("error in (no error)"=w859, "Python Object References In"=w862, "Session ID"=w865) -> ("error out"=w858:errorcluster, "Value"=→"Flow 9":dbl, "Python Object References Out"=w861:T5, "Session ID out"=w864:T4)  [unwired: 5 in]
                n224 = call-poly <vilib>:"Unpack.vi"("error in (no error)"=w858, "Python Object References In"=w861, "Session ID"=w864) -> ("error out"=w852:errorcluster, "Value"=→"Conc 9":dbl, "Python Object References Out"=w853:T5, "Session ID out"=w854:T4)  [unwired: 5 in]
                n225 = call-poly <vilib>:"Unpack.vi"("error in (no error)"=w852, "Python Object References In"=w853, "Session ID"=w854) -> ("error out"=w904:errorcluster, "Value"=→"Param 1 8":dbl, "Python Object References Out"=w902:T5, "Session ID out"=w900:T4)  [unwired: 5 in]
                n226 = call-poly <vilib>:"Unpack.vi"("error in (no error)"=w904, "Python Object References In"=w902, "Session ID"=w900) -> ("error out"=w905:errorcluster, "Value"=→"T value 1 8":dbl, "Python Object References Out"=w903:T5, "Session ID out"=w901:T4)  [unwired: 5 in]
                n227 = call-poly <vilib>:"Unpack.vi"("error in (no error)"=w905, "Python Object References In"=w903, "Session ID"=w901) -> ("error out"=w906:errorcluster, "Value"=→"Param 2 8":dbl, "Python Object References Out"=w897:T5, "Session ID out"=w896:T4)  [unwired: 5 in]
                n228 = call-poly <vilib>:"Unpack.vi"("error in (no error)"=w906, "Python Object References In"=w897, "Session ID"=w896) -> ("error out"=w888:errorcluster, "Value"=→"T value 2 8":dbl, "Python Object References Out"=w890:T5, "Session ID out"=w892:T4)  [unwired: 5 in]
                n229 = call-poly <vilib>:"Unpack.vi"("error in (no error)"=w888, "Python Object References In"=w890, "Session ID"=w892) -> ("error out"=w887:errorcluster, "Value"=→"T Ref 8":dbl, "Python Object References Out"=w889:T5, "Session ID out"=w891:T4)  [unwired: 5 in]
                n230 = call-poly <vilib>:"Unpack.vi"("error in (no error)"=w887, "Python Object References In"=w889, "Session ID"=w891) -> ("error out"=w870:errorcluster, "Value"=→"Correlation 8":dbl, "Python Object References Out"=w871:T5, "Session ID out"=w872:T4)  [unwired: 5 in]
                n231 = call-poly <vilib>:"Unpack.vi"("error in (no error)"=w870, "Python Object References In"=w871, "Session ID"=w872) -> ("error out"=w884:errorcluster, "Value"=→"X2 8":dbl, "Python Object References Out"=w883:T5, "Session ID out"=w882:T4)  [unwired: 5 in]
                n232 = call-poly <vilib>:"Unpack.vi"("error in (no error)"=w884, "Python Object References In"=w883, "Session ID"=w882) -> ("error out"=w867:errorcluster, "Value"=→"X2 ref 8":dbl, "Session ID out"=w868:T4)  [unwired: 5 in, 1 out]
                n233 = call <vilib>:"Close Session.vi"("error in (no error)"=w867, "Session ID"=w868) -> ()  [unwired: 9 in, 1 out]
              }
            }
            "Exp 9" <- TRUE
          }
        }
      }
      frame True {
        w911 = 0
      }
    }
    n234 = timed-loop {
      tunnel: w124 -> [w1065]
      tunnel: w123 -> [w1064]
      tunnel: [w1013] -> w122
      tunnel: [w1012] -> w121
      timing: w120 -> [_]
      timing-out: [_] -> w119
      tunnel: w118 -> [w999]
      tunnel: w117 -> [w1003]
      tunnel: w116 -> [w1002]
      tunnel: [w998] -> w115
      tunnel: [w997] -> w114
      tunnel: [w978] -> w113
      tunnel: w104 -> [w994]
      tunnel: w103 -> [w916]
      tunnel: w102 -> [w935]
      tunnel: w112 -> [w983]
      tunnel: w111 -> [w982]
      tunnel: w110 -> [w981]
      tunnel: w109 -> [w980]
      shift-right: [w940] -> _
      shift-left: _ -> [w972]
      tunnel: [w975] -> w108
      tunnel: [w974] -> w107
      tunnel: ["Stop everything"] -> w105
      tunnel: "Automated Experiments or Direct Control" -> [w941]
      tunnel: w91 -> [w930]
      tunnel: w90 -> [w929]
      tunnel: [w928] -> w89
      tunnel: [w927] -> w88
      i -> [w963]
      stop <- w970 stop-if-true
      w979 = 9.0 ("Safety Shut Down Pressure (barg)")
      w995 = 180
      # "in case out of range changes conc to within possible range"
      # "1st 4 flowrates\n5,6 temperatures\n7 pressure (1)\n8 gas (1)"
      # "temperature or syringe or pressure"
      # "We are graphing in barg"
      # "temperature or syringe"
      # "Empty Syringe has level of 50"
      n235 = node-c288() -> ()  [unwired: 1 in, 1 out]
      n236 = call-poly <vilib>:"DAQmx Read.vi"("task/channels in"=w930, "error in"=w929) -> ("task out"=w928:refnum<k21>, "data"=w923:dbl, "error out"=w927:errorcluster)  [unwired: 11 in]
      n237 = Multiply(x=5.1522, y=w923) -> (x*y=w926:dbl)
      n238 = Add(x=-2.6852, y=w926) -> (x+y=w919:dbl)
      "Liquid Inlet Pressure (bar g)" <- w919
      n239 = Greater?(x=w916, y=50) -> (0:w917:bool)
      n240 = Less?(x=w916, y=0) -> (x < y?=w914:bool)
      n241 = case shown="False" w917 {
        tunnel: [w1069 1] -> w913
        tunnel: w916 -> [w1069 _]
        frame False {
        }
        frame True {
        }
      }
      n242 = case shown="False" w914 {
        tunnel: [w1067 1] -> w912
        tunnel: w913 -> [w1067 _]
        frame False {
        }
        frame True {
        }
      }
      n243 = for {
        N: 4 -> [_]
        tunnel: w1065 -> [w1346] mode=indexing
        tunnel: [w1344] -> w1059 mode=indexing
        tunnel: [w1341] -> w1054 mode=indexing
        tunnel: [w1340] -> w1053 mode=indexing
        tunnel: [w1339] -> w1052 mode=indexing
        tunnel: w1064 -> [w1338] mode=indexing
        i -> [w1345]
        n244 = call "NCS_GetFlowRateIs.vi"("error in (no error)"=w1338, "dosingunit"=w1345, "device handle in"=w1346) -> ("error out"=w1342:errorcluster, "flowrate is"=w1344:dbl, "device handle out"=w1343:u32)
        n245 = call "NCS_GetSyringeLevelIs.vi"("error in (no error)"=w1342, "dosingunit"=w1345, "device handle in"=w1343) -> ("error out"=w1339:errorcluster, "syringe level is"=w1341:dbl, "device handle out"=w1340:u32)
      }
      n246 = Index Array(array=w1054, index=0) -> (element=w967:dbl)
      "Syringe Level 1" <- w967
      n247 = Index Array(array=w1054, index=3) -> (element=w964:dbl)
      "Syringe Level 4" <- w964
      n248 = Index Array(array=w1054, index=1) -> (element=w966:dbl)
      "Syringe Level 2" <- w966
      n249 = Index Array(array=w1054, index=2) -> (element=w965:dbl)
      "Syringe Level 3" <- w965
      n250 = case shown="True" "Shut down in empty?\nLeft off, right on" {
        tunnel: [FALSE w1240] -> w968
        tunnel: w967 -> [_ w1239]
        tunnel: w966 -> [_ w1238]
        tunnel: w965 -> [_ w1237]
        tunnel: w964 -> [_ w1236]
        frame False {
        }
        frame True {
          w1241 = 50
          n251 = Less Or Equal?(x=w1238, y=w1241) -> (x <= y?=w1247:bool)
          n252 = Less Or Equal?(x=w1239, y=w1241) -> (x <= y?=w1242:bool)
          n253 = Less Or Equal?(x=w1237, y=w1241) -> (x <= y?=w1245:bool)
          n254 = Less Or Equal?(x=w1236, y=w1241) -> (x <= y?=w1243:bool)
          n255 = Or(x=w1242, y=w1247) -> (x .or. y?=w1246:bool)
          n256 = Or(x=w1246, y=w1245) -> (x .or. y?=w1244:bool)
          n257 = Or(x=w1244, y=w1243) -> (x .or. y?=w1240:bool)
        }
      }
      n258 = Index Array(array=w1059, index=0) -> (element=w951:dbl)
      "Flowrate 1 Low" <- w951
      n259 = Index Array(array=w1059, index=3) -> (element=w953:dbl)
      "Flowrate 4 Ethanol" <- w953
      n260 = Index Array(array=w1059, index=1) -> (element=w950:dbl)
      "Flowrate 2 High" <- w950
      n261 = Index Array(array=w1059, index=2) -> (element=w954:dbl)
      "Flowrate 3 Acid" <- w954
      n262 = case shown="True" "Clear" {
        tunnel: w972 -> [w1248 _]
        tunnel: [w1248 w1249] -> w971
        frame False {
        }
        frame True {
          n263 = Initialize Array(0, 1) -> (w1249:i32[])
        }
      }
      n264 = call-poly <vilib>:"DAQmx Read.vi"("task/channels in"=w983, "error in"=w982) -> ("task out"=w975:refnum<k21>, "data"=w988:dbl[], "error out"=w974:errorcluster)  [unwired: 11 in]
      n265 = Add(x=w951, y=w950) -> (x+y=w956:dbl)
      n266 = Add(x=w956, y=w954) -> (x+y=w955:dbl)
      n267 = Index Array(array=w988, index=0) -> (element=w986:dbl)
      n268 = Add(x=w955, y=w953) -> (x+y=w952:dbl)
      "Total Flowrate (uL/min)" <- w952
      n269 = Divide(x=w951, y=w952) -> (x/y=w945:dbl)
      n270 = Multiply(x=w986, y=w981) -> (x*y=w987:dbl)
      n271 = Multiply(x="Low Conc", y=w945) -> (x*y=w949:dbl)
      n272 = Add(x=w987, y=w980) -> (x+y=w984:dbl)
      n273 = Divide(x=w950, y=w952) -> (x/y=w946:dbl)
      n274 = Multiply(x="High Conc", y=0.9) -> (x*y=w937:dbl)
      n275 = Multiply(x="Low Conc", y=0.9) -> (x*y=w936:dbl)
      n276 = Multiply(x="High Conc", y=w946) -> (x*y=w948:dbl)
      n277 = Add(x=w949, y=w948) -> (x+y=→"Feed Concentration (M)":dbl)
      n278 = In Range and Coerce(upper limit=w937, x=w935, lower limit=w936) -> (coerced(x)=w932:dbl, In Range?=w934:bool)
      n279 = case shown="True" w934 {
        tunnel: [w1072 w1074] -> w933
        tunnel: w935 -> [_ w1074]
        tunnel: w932 -> [w1072 _]
        tunnel: [TRUE FALSE] -> w931
        frame False {
        }
        frame True {
        }
      }
      "Desired Conc Not Possible" <- w931
      n280 = Multiply(x=w984, y=0.0689476) -> (x*y=w920:dbl)
      "Gas Back Pressure (barg)" <- w920
      n281 = case shown="False" w941 {
        tunnel: [w1318 w1319] -> w1050
        tunnel: w912 -> [w1305 _]
        tunnel: w933 -> [w1307 _]
        tunnel: "High Conc" -> [w1304 _]
        tunnel: "Low Conc" -> [w1303 _]
        frame False {
          w1302 = 0.1
          # "swapped it so syringe 2 is high and 1 is low"
          n282 = Subtract(x=w1304, y=w1303) -> (x-y=w1314:dbl)
          n283 = Subtract(x=1, y=w1302) -> (x-y=w1310:dbl)
          n284 = Divide(x=w1307, y=w1310) -> (x/y=w1316:dbl)
          n285 = Multiply(x=0, y=w1305) -> (x*y=w1300:dbl)
          n286 = Subtract(x=w1304, y=w1316) -> (x-y=w1313:dbl)
          n287 = Subtract(x=w1316, y=w1303) -> (x-y=w1315:dbl)
          n288 = Divide(x=w1315, y=w1314) -> (x/y=w1312:dbl)
          n289 = Divide(x=w1313, y=w1314) -> (x/y=w1311:dbl)
          n290 = Multiply(x=w1312, y=w1310) -> (x*y=w1309:dbl)
          n291 = Multiply(x=w1311, y=w1310) -> (x*y=w1308:dbl)
          n292 = Multiply(x=w1305, y=w1308) -> (x*y=w1298:dbl)
          n293 = Multiply(x=w1305, y=w1309) -> (x*y=w1299:dbl)
          n294 = Multiply(x=w1305, y=w1302) -> (x*y=w1301:dbl)
          n295 = Build Array(w1298, w1299, w1301, w1300) -> (w1318:dbl[])
          "Volumetric Fraction Acid" <- w1302
        }
        frame True {
          n296 = Build Array("Set Flowrate 1", "Set Flowrate 2", "Set Flowrate 3", "Set Flowrate 4") -> (w1319:dbl[])
        }
      }
      n297 = Build Array (concatenate)(w971, w920) -> (w940:dbl[])
      "Calculated Pressure" <- w940
      n298 = Greater Or Equal?(x=w920, y=w979) -> (x >= y?=w976:bool)
      n299 = case shown="True" w941 {
        tunnel: [w1253 FALSE] -> w943
        tunnel: w963 -> [w1252 _]
        frame False {
          # "changes set points for each new exp"
          n300 = Equal?(x=w1252, y=0) -> (x = y?=w1253:bool)
        }
        frame True {
          # "at end of each exp"
          # "doesnt automatically change set point"
        }
      }
      n301 = Or(x=w943, y="Update Temperature Set Point") -> (x .or. y?=w1005:bool)
      n302 = case shown="True" w1005 {
        tunnel: w1003 -> [w1257 w1265]
        tunnel: w1002 -> [w1256 w1264]
        tunnel: [w1257 w1263] -> w1001
        tunnel: [w1256 w1262] -> w1000
        tunnel: w999 -> [_ w1261]
        tunnel: w941 -> [_ w1259]
        tunnel: w994 -> [_ w1258]
        frame False {
        }
        frame True {
          n303 = case shown="True" w1259 {
            tunnel: [w1266 "Set Point (oC)"] -> w1260
            tunnel: w1258 -> [w1266 _]
            frame False {
            }
            frame True {
            }
          }
          n304 = call "CN7500_Write Set Point Value.vi"("Target Set Point Value"=w1260, "error in (no error)"=w1264, "Controller Number"=w1261, "VISA In"=w1265) -> ("error out"=w1262:errorcluster, "VISA Out"=w1263:refnum<visa-resource-name>)  [unwired: 6 in]
        }
      }
      n305 = Or(x="Generate Flow", y=w943) -> (x .or. y?=w944:bool)
      n306 = case shown="True" w944 {
        tunnel: w1053 -> [w1325 w1330]
        tunnel: w1052 -> [w1324 w1329]
        tunnel: [w1324 w1328] -> w958
        tunnel: [w1325 w1327] -> w957
        tunnel: w1050 -> [_ w1326]
        frame False {
        }
        frame True {
          n307 = for {
            N: 4 -> [_]
            tunnel: w1330 -> [w1337] mode=indexing
            tunnel: w1329 -> [w1336] mode=indexing
            tunnel: [w1335] -> w1328 mode=indexing
            tunnel: [w1334] -> w1327 mode=indexing
            tunnel: w1326 -> [w1332] mode=indexing
            i -> [w1333]
            n308 = call "NCS_GenerateFlow.vi"("error in (no error)"=w1336, "flowrate"=w1332, "dosingunit"=w1333, "device handle in"=w1337) -> ("error out"=w1335:errorcluster, "device handle out"=w1334:u32)
          }
        }
      }
      n309 = call "CN7500_Read Process Value.vi"("error in (no error)"=w1000, "Controller Number"=w999, "VISA In"=w1001) -> ("error out"=w998:errorcluster, "Set Point Value"=w990:dbl, "Process Value"=w991:dbl, "VISA Out"=w997:refnum<visa-resource-name>)  [unwired: 5 in]
      "Temp Set Point (oC)" <- w990
      "Actual Temp (oC)" <- w991
      n310 = Merge Signals(w991, w990) -> (→"Temperature":dynamicdata)
      n311 = Merge Signals(w951, w950, w954, w953, w991, w990, w920, w919) -> (w1011:dynamicdata)
      n312 = Greater Or Equal?(x=w991, y=w995) -> (x >= y?=w993:bool)
      n313 = call "Write To Measurement File"("Signals"=w1011) -> ()  [unwired: 16 in, 3 out]
      n314 = Index Array(array=w958, index=0) -> (element=w1040:errorcluster)
      n315 = Index Array(array=w957, index=0) -> (element=w1041:u32)
      n316 = Index Array(array=w958, index=3) -> (element=w1030:errorcluster)
      n317 = Index Array(array=w958, index=2) -> (element=w1032:errorcluster)
      n318 = Index Array(array=w958, index=1) -> (element=w1034:errorcluster)
      n319 = Index Array(array=w957, index=3) -> (element=w1031:u32)
      n320 = Index Array(array=w957, index=2) -> (element=w1033:u32)
      n321 = Index Array(array=w957, index=1) -> (element=w1035:u32)
      n322 = case shown="False" "Stop Dose 2" {
        tunnel: w1035 -> [w1285 w1290]
        tunnel: w1034 -> [w1284 w1289]
        tunnel: [w1285 w1288] -> w1027
        tunnel: [w1284 w1287] -> w1026
        frame False {
        }
        frame True {
          n323 = call "NCS_Stop.vi"("error in (no error)"=w1289, "dosingunit"=1, "device handle in"=w1290) -> ("error out"=w1287:errorcluster, "device handle out"=w1288:u32)
        }
      }
      n324 = case shown="False" "Stop Dose 1" {
        tunnel: w1041 -> [w1292 w1297]
        tunnel: w1040 -> [w1291 w1296]
        tunnel: [w1292 w1295] -> w1029
        tunnel: [w1291 w1294] -> w1028
        frame False {
        }
        frame True {
          n325 = call "NCS_Stop.vi"("error in (no error)"=w1296, "dosingunit"=0, "device handle in"=w1297) -> ("error out"=w1294:errorcluster, "device handle out"=w1295:u32)
        }
      }
      n326 = case shown="False" "Stop Dose 3" {
        tunnel: w1033 -> [w1278 w1283]
        tunnel: w1032 -> [w1277 w1282]
        tunnel: [w1278 w1281] -> w1025
        tunnel: [w1277 w1280] -> w1024
        frame False {
        }
        frame True {
          n327 = call "NCS_Stop.vi"("error in (no error)"=w1282, "dosingunit"=2, "device handle in"=w1283) -> ("error out"=w1280:errorcluster, "device handle out"=w1281:u32)
        }
      }
      n328 = case shown="False" "Stop Dose 4" {
        tunnel: w1031 -> [w1271 w1276]
        tunnel: w1030 -> [w1270 w1275]
        tunnel: [w1271 w1274] -> w1023
        tunnel: [w1270 w1273] -> w1022
        frame False {
        }
        frame True {
          n329 = call "NCS_Stop.vi"("error in (no error)"=w1275, "dosingunit"=3, "device handle in"=w1276) -> ("error out"=w1273:errorcluster, "device handle out"=w1274:u32)
        }
      }
      n330 = case shown="False" "Safety or Emergency Syringe Control" {
        tunnel: w1029 -> [w1082 w1123]
        tunnel: w1028 -> [w1078 w1122]
        tunnel: w1027 -> [w1081 w1121]
        tunnel: w1026 -> [w1077 w1120]
        tunnel: w1025 -> [w1080 w1119]
        tunnel: w1024 -> [w1076 w1118]
        tunnel: w1023 -> [w1079 w1117]
        tunnel: w1022 -> [w1075 w1116]
        tunnel: [w1082 w1093] -> w1021
        tunnel: [w1081 w1092] -> w1020
        tunnel: [w1080 w1091] -> w1019
        tunnel: [w1079 w1090] -> w1018
        tunnel: [w1077 w1089] -> w1017
        tunnel: [w1076 w1088] -> w1016
        tunnel: [w1075 w1087] -> w1015
        tunnel: [w1078 w1083] -> w1014
        frame False {
        }
        frame True {
          n331 = case shown="False" "Calibrate 2" {
            tunnel: w1121 -> [w1222 w1227]
            tunnel: w1120 -> [w1221 w1226]
            tunnel: [w1222 w1225] -> w1110
            tunnel: [w1221 w1224] -> w1109
            frame False {
            }
            frame True {
              n332 = call "NCS_Calibrate.vi"("error in (no error)"=w1226, "dosingunit"=1, "device handle in"=w1227) -> ("error out"=w1224:errorcluster, "device handle out"=w1225:u32)
            }
          }
          n333 = case shown="False" "Calibrate 3" {
            tunnel: w1119 -> [w1215 w1220]
            tunnel: w1118 -> [w1214 w1219]
            tunnel: [w1215 w1218] -> w1108
            tunnel: [w1214 w1217] -> w1107
            frame False {
            }
            frame True {
              n334 = call "NCS_Calibrate.vi"("error in (no error)"=w1219, "dosingunit"=2, "device handle in"=w1220) -> ("error out"=w1217:errorcluster, "device handle out"=w1218:u32)
            }
          }
          n335 = case shown="False" "Calibrate 1" {
            tunnel: w1123 -> [w1229 w1234]
            tunnel: w1122 -> [w1228 w1233]
            tunnel: [w1229 w1232] -> w1112
            tunnel: [w1228 w1231] -> w1111
            frame False {
            }
            frame True {
              n336 = call "NCS_Calibrate.vi"("error in (no error)"=w1233, "dosingunit"=0, "device handle in"=w1234) -> ("error out"=w1231:errorcluster, "device handle out"=w1232:u32)
            }
          }
          n337 = case shown="False" "Calibrate 4" {
            tunnel: w1117 -> [w1208 w1213]
            tunnel: w1116 -> [w1207 w1212]
            tunnel: [w1208 w1211] -> w1106
            tunnel: [w1207 w1210] -> w1105
            frame False {
            }
            frame True {
              n338 = call "NCS_Calibrate.vi"("error in (no error)"=w1212, "dosingunit"=3, "device handle in"=w1213) -> ("error out"=w1210:errorcluster, "device handle out"=w1211:u32)
            }
          }
          n339 = case shown="False" "Empty 2" {
            tunnel: w1110 -> [w1188 w1192]
            tunnel: w1109 -> [w1187 w1190]
            tunnel: [w1188 w1191] -> w1096
            tunnel: [w1187 w1189] -> w1097
            frame False {
            }
            frame True {
              w1194 = 1
              n340 = call "NCS_GetFlowRateMax.vi"("error in (no error)"=w1190, "dosingunit"=w1194, "device handle in"=w1192) -> ("error out"=w1195:errorcluster, "flow rate max"=w1193:dbl, "device handle out"=w1196:u32)
              n341 = call "NCS_EmptySyrige.vi"("error in (no error)"=w1195, "flowrate"=w1193, "dosingunit"=w1194, "device handle in"=w1196) -> ("error out"=w1189:errorcluster, "device handle out"=w1191:u32)
            }
          }
          n342 = case shown="False" "Empty 1" {
            tunnel: w1112 -> [w1198 w1206]
            tunnel: w1111 -> [w1197 w1203]
            tunnel: [w1198 w1204] -> w1094
            tunnel: [w1197 w1201] -> w1095
            frame False {
            }
            frame True {
              w1200 = 0
              n343 = call "NCS_GetFlowRateMax.vi"("error in (no error)"=w1203, "dosingunit"=w1200, "device handle in"=w1206) -> ("error out"=w1202:errorcluster, "flow rate max"=w1199:dbl, "device handle out"=w1205:u32)
              n344 = call "NCS_EmptySyrige.vi"("error in (no error)"=w1202, "flowrate"=w1199, "dosingunit"=w1200, "device handle in"=w1205) -> ("error out"=w1201:errorcluster, "device handle out"=w1204:u32)
            }
          }
          n345 = case shown="False" "Empty 3" {
            tunnel: w1108 -> [w1178 w1179]
            tunnel: w1107 -> [w1177 w1180]
            tunnel: [w1178 w1181] -> w1098
            tunnel: [w1177 w1182] -> w1099
            frame False {
            }
            frame True {
              w1184 = 2
              n346 = call "NCS_GetFlowRateMax.vi"("error in (no error)"=w1180, "dosingunit"=w1184, "device handle in"=w1179) -> ("error out"=w1185:errorcluster, "flow rate max"=w1183:dbl, "device handle out"=w1186:u32)
              n347 = call "NCS_EmptySyrige.vi"("error in (no error)"=w1185, "flowrate"=w1183, "dosingunit"=w1184, "device handle in"=w1186) -> ("error out"=w1182:errorcluster, "device handle out"=w1181:u32)
            }
          }
          n348 = case shown="False" "Empty 4" {
            tunnel: w1106 -> [w1168 w1169]
            tunnel: w1105 -> [w1167 w1170]
            tunnel: [w1168 w1172] -> w1100
            tunnel: [w1167 w1171] -> w1101
            frame False {
            }
            frame True {
              w1174 = 3
              n349 = call "NCS_GetFlowRateMax.vi"("error in (no error)"=w1170, "dosingunit"=w1174, "device handle in"=w1169) -> ("error out"=w1175:errorcluster, "flow rate max"=w1173:dbl, "device handle out"=w1176:u32)
              n350 = call "NCS_EmptySyrige.vi"("error in (no error)"=w1175, "flowrate"=w1173, "dosingunit"=w1174, "device handle in"=w1176) -> ("error out"=w1171:errorcluster, "device handle out"=w1172:u32)
            }
          }
          n351 = case shown="False" "Refill 2" {
            tunnel: w1096 -> [w1148 w1152]
            tunnel: w1097 -> [w1147 w1150]
            tunnel: [w1148 w1151] -> w1092
            tunnel: [w1147 w1149] -> w1089
            frame False {
            }
            frame True {
              w1154 = 1
              n352 = call "NCS_GetFlowRateMax.vi"("error in (no error)"=w1150, "dosingunit"=w1154, "device handle in"=w1152) -> ("error out"=w1155:errorcluster, "flow rate max"=w1153:dbl, "device handle out"=w1156:u32)
              n353 = call "NCS_RefillSyrige.vi"("error in (no error)"=w1155, "flowrate"=w1153, "dosingunit"=w1154, "device handle in"=w1156) -> ("error out"=w1149:errorcluster, "device handle out"=w1151:u32)
            }
          }
          n354 = case shown="False" "Refill 1" {
            tunnel: w1094 -> [w1158 w1166]
            tunnel: w1095 -> [w1157 w1163]
            tunnel: [w1158 w1164] -> w1093
            tunnel: [w1157 w1161] -> w1083
            frame False {
            }
            frame True {
              w1160 = 0
              n355 = call "NCS_GetFlowRateMax.vi"("error in (no error)"=w1163, "dosingunit"=w1160, "device handle in"=w1166) -> ("error out"=w1162:errorcluster, "flow rate max"=w1159:dbl, "device handle out"=w1165:u32)
              n356 = call "NCS_RefillSyrige.vi"("error in (no error)"=w1162, "flowrate"=w1159, "dosingunit"=w1160, "device handle in"=w1165) -> ("error out"=w1161:errorcluster, "device handle out"=w1164:u32)
            }
          }
          n357 = case shown="False" "Refill 3" {
            tunnel: w1098 -> [w1138 w1139]
            tunnel: w1099 -> [w1137 w1140]
            tunnel: [w1138 w1141] -> w1091
            tunnel: [w1137 w1142] -> w1088
            frame False {
            }
            frame True {
              w1144 = 2
              n358 = call "NCS_GetFlowRateMax.vi"("error in (no error)"=w1140, "dosingunit"=w1144, "device handle in"=w1139) -> ("error out"=w1145:errorcluster, "flow rate max"=w1143:dbl, "device handle out"=w1146:u32)
              n359 = call "NCS_RefillSyrige.vi"("error in (no error)"=w1145, "flowrate"=w1143, "dosingunit"=w1144, "device handle in"=w1146) -> ("error out"=w1142:errorcluster, "device handle out"=w1141:u32)
            }
          }
          n360 = case shown="False" "Refill 4" {
            tunnel: w1100 -> [w1128 w1129]
            tunnel: w1101 -> [w1127 w1130]
            tunnel: [w1128 w1132] -> w1090
            tunnel: [w1127 w1131] -> w1087
            frame False {
            }
            frame True {
              w1134 = 3
              n361 = call "NCS_GetFlowRateMax.vi"("error in (no error)"=w1130, "dosingunit"=w1134, "device handle in"=w1129) -> ("error out"=w1135:errorcluster, "flow rate max"=w1133:dbl, "device handle out"=w1136:u32)
              n362 = call "NCS_RefillSyrige.vi"("error in (no error)"=w1135, "flowrate"=w1133, "dosingunit"=w1134, "device handle in"=w1136) -> ("error out"=w1131:errorcluster, "device handle out"=w1132:u32)
            }
          }
        }
      }
      n363 = Or(x=w993, y=w968) -> (x .or. y?=w977:bool)
      n364 = Or(x=w977, y=w976) -> (x .or. y?=w978:bool)
      n365 = Multiply(x="Minutes between Exp", y=60) -> (x*y=w960:dbl)
      n366 = Divide(x=w960, y=5) -> (x/y=w961:dbl)
      n367 = Greater Or Equal?(x=w963, y=w961) -> (x >= y?=w1007:bool)
      n368 = Or(x=w1007, y=w978) -> (x .or. y?=w992:bool)
      n369 = Or(x="Skip Exp", y=w992) -> (x .or. y?=w1008:bool)
      n370 = Or(x="Stop everything", y=w1008) -> (x .or. y?=w970:bool)
      n371 = node-c288() -> ()  [unwired: 1 in, 1 out]
      n372 = Build Array(w1021, w1020, w1019, w1018) -> (w1013:u32[])
      n373 = Build Array(w1014, w1017, w1016, w1015) -> (w1012:errorcluster[])
      "loop ind" <- w963
      "Safety Shut Down Temp" <- w995
      "Safety Shut Down Pressure (barg)" <- w979
    }
    n374 = Or(x=w105, y=w113) -> (x .or. y?=w106:bool)
    n375 = node-c288(w119) -> ()  [unwired: 1 out]
  }
  n376 = call <vilib>:"DAQmx Stop Task.vi"("task/channels in"=w16, "error in"=w15) -> ("task out"=w18:refnum<k21>, "error out"=w17:errorcluster)  [unwired: 12 in]
  n377 = Index Array(array=w45, index=0) -> (element=w47:u32)
  n378 = Index Array(array=w44, index=0) -> (element=w46:errorcluster)
  n379 = call <vilib>:"DAQmx Stop Task.vi"("task/channels in"=w5, "error in"=w3) -> ("task out"=w4:refnum<k21>, "error out"=w6:errorcluster)  [unwired: 12 in]
  n380 = call <vilib>:"DAQmx Clear Task.vi"("task in"=w18, "error in"=w17) -> ()  [unwired: 13 in, 1 out]
  n381 = call <vilib>:"DAQmx Clear Task.vi"("task in"=w4, "error in"=w6) -> ()  [unwired: 13 in, 1 out]
  n382 = call "NCS_CloseDevice.vi"("error in (no error)"=w46, "device handle"=w47) -> ()  [unwired: 1 out]
  n383 = call "CN7500_Write Set Point Value.vi"("Target Set Point Value"=25, "error in (no error)"=w33, "Controller Number"=w36, "VISA In"=w32) -> ("error out"=w38:errorcluster, "VISA Out"=w39:refnum<visa-resource-name>)  [unwired: 6 in]
  n384 = call "CN7500_Close.vi"("error in (no error)"=w38, "VISA resource name"=w39) -> ()  [unwired: 9 in, 1 out]
